vi "FTW-Test-SQLite-BasicQuery.vi"() -> (0 "Test Result":errorcluster)   [LabVIEW 2014]
uses:
  src/core/database/FTW-SQLite-DatabaseType.ctl
  src/core/time/FTW-Time-Uptime.vi
  src/core/error/FTW-ERR-Assert-DeveloperError.vi
  src/core/error/FTW-ERR-ThrowError.vi
  src/core/error/FTW-ERR-NoErrorConstant.vi
  src/core/database/FTW-SQLite-PrepareStatement.vi
  src/core/database/FTW-SQLite-LibraryReturnValue.vi
  src/core/error/FTW-ERR-CallChain.vi
  src/core/string/FTW-STR-ReplaceWhitespace.vi
  src/core/database/FTW-SQLite-Insert/FTW-SQLite-Insert.xnode
  src/core/database/FTW-SQLite-Connector.lvclass
  src/core/database/FTW-SQLite-Fetch/FTW-SQLite-Fetch.xnode
  src/core/database/FTW-SQLite-AccessMode.ctl
panel:
  out "Results from Database":T1(array[cluster])
  out "Data to put into Database":T2(array[cluster])
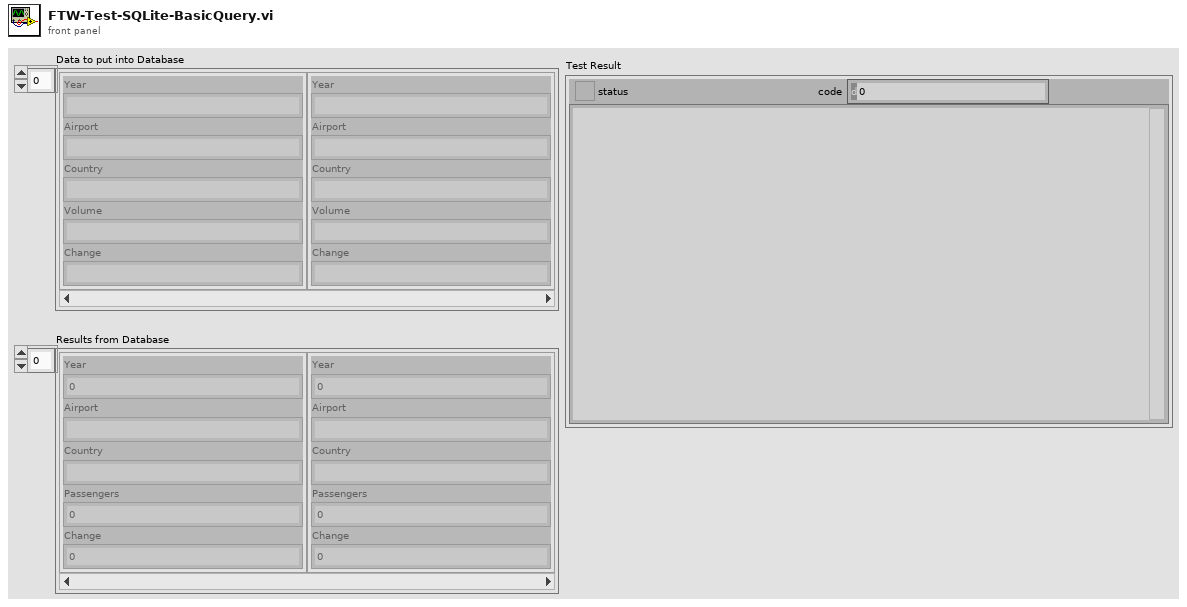
[diagram p1: front panel]
types:
  T1 = cluster{"Year":i32, "Airport":string, "Country":string, "Passengers":i32, "Change":dbl}[]
  T2 = cluster{"Year":string, "Airport":string, "Country":string, "Volume":string, "Change":string}[]
  T3 = cluster{"Year":string, "Airport":string, "Country":string, "Volume":string, "Change":string}
  T4 = cluster{"Year":i32, "Airport":string, "Country":string, "Passengers":i32, "Change":dbl}
  T5 = typedef "FTW-SQLite-Connector.lvclass/FTW-SQLite-DatabaseType.ctl" = enum16{"Disk", "Memory"}
  T6 = typedef "FTW-SQLite-Connector.lvclass/FTW-SQLite-AccessMode.ctl" = enum16{"Read", "Read/Write", "Read/Write/Create"}
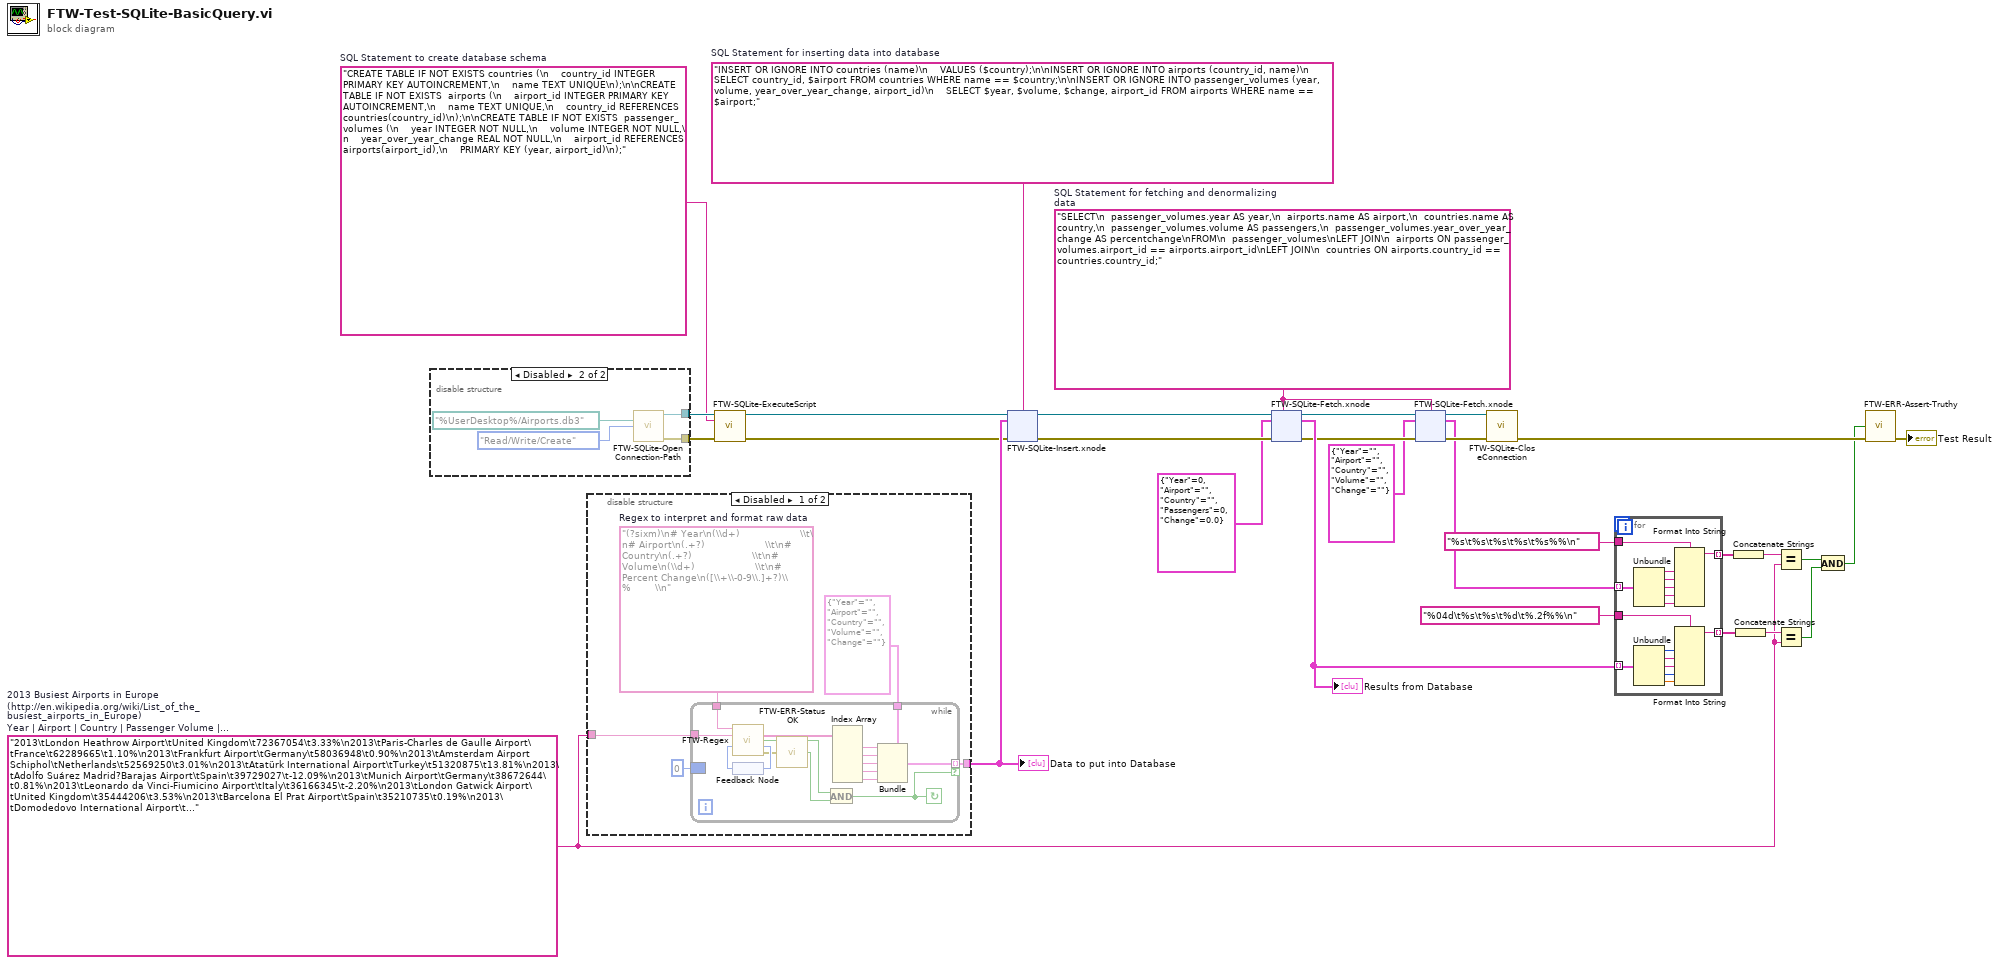
[diagram p0: block diagram]
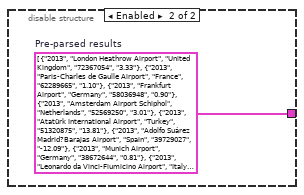
[diagram p2: hidden frame]
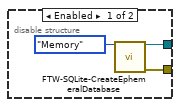
[diagram p3: hidden frame]
diagram:
  w23 = "INSERT OR IGNORE INTO countries (name)\n    VALUES ($country);\n\nINSERT OR IGNORE INTO airports (country_id, name)\n    SELECT country_id, $airport FROM countries WHERE name == $country;\n\nINSERT OR IGNORE INTO passenger_volumes (year, volume, year_over_year_change, airport_id)\n    SELECT $year, $volume, $change, airport_id FROM airports WHERE name == $airport;"  # SQL Statement for inserting data into database
  w10 = "SELECT\n  passenger_volumes.year AS year,\n  airports.name AS airport,\n  countries.name AS country,\n  passenger_volumes.volume AS passengers,\n  passenger_volumes.year_over_year_change AS percentchange\nFROM\n  passenger_volumes\nLEFT JOIN\n  airports ON passenger_volumes.airport_id == airports.airport_id\nLEFT JOIN\n  countries ON airports.country_id == countries.country_id;"  # SQL Statement for fetching and denormalizing data
  w2 = "2013\tLondon Heathrow Airport\tUnited Kingdom\t72367054\t3.33%\n2013\tParis-Charles de Gaulle Airport\tFrance\t62289665\t1.10%\n2013\tFrankfurt Airport\tGermany\t58036948\t0.90%\n2013\tAmsterdam Airport Schiphol\tNetherlands\t52569250\t3.01%\n2013\tAtatürk International Airport\tTurkey\t51320875\t13.81%\n2013\tAdolfo Suárez Madrid?Barajas Airport\tSpain\t39729027\t-12.09%\n2013\tMunich Airport\tGermany\t38672644\t0.81%\n2013\tLeonardo da Vinci-Fiumicino Airport\tItaly\t36166345\t-2.20%\n2013\tLondon Gatwick Airport\tUnited Kingdom\t35444206\t3.53%\n2013\tBarcelona El Prat Airport\tSpain\t35210735\t0.19%\n2013\tDomodedovo International Airport\tRussia\t30760000\t9.21%\n2013\tSheremetyevo International Airport\tRussia\t29256000\t12.38%\n2013\tParis-Orly Airport\tFrance\t28274154\t3.83%\n2013\tAntalya Airport\tTurkey\t27003712\t8.04%\n2013\tZürich Airport\tSwitzerland\t24865138\t0.25%\n2013\tCopenhagen Airport, Kastrup\tDenmark\t24067030\t3.13%\n2013\tOslo Gardermoen International Airport\tNorway\t22956540\t3.97%\n2013\tPalma de Mallorca Airport\tSpain\t22768082\t0.45%\n2013\tVienna International Airport\tAustria\t21999926\t-0.75%\n2013\tDüsseldorf International Airport\tGermany\t21228226\t1.90%\n2013\tManchester Airport\tUnited Kingdom\t20751581\t5.14%\n2013\tStockholm-Arlanda Airport\tSweden\t20681554\t5.29%\n2013\tDublin Airport\tIreland\t20200000\t5.76%\n2013\tBerlin Tegel Airport\tGermany\t19591838\t7.86%\n2013\tBrussels Airport\tBelgium\t19133222\t0.85%\n2013\tSabiha Gökçen Airport\tTurkey\t18641842\t28.68%\n2013\tMalpensa Airport\tItaly\t17955075\t-3.14%\n2013\tLondon Stansted Airport\tUnited Kingdom\t17852393\t2.17%\n2013\tLisbon Portela Airport\tPortugal\t16024955\t4.73%\n2013\tHelsinki-Vantaa Airport\tFinland\t15279043\t2.83%\n2013\tGeneva International Airport\tSwitzerland\t14436149\t3.86%\n2013\tHamburg Airport\tGermany\t13502553\t-1.42%\n2013\tMálaga Airport\tSpain\t12922403\t2.71%\n2013\tPulkovo Airport\tRussia\t12854366\t15.24%\n2013\tAthens International Airport\tGreece\t12460298\t-3.74%\n2013\tNice Côte d'Azur Airport\tFrance\t11554195\t3.26%\n2013\tVnukovo International Airport\tRussia\t11180000\t15.38%\n2013\tVáclav Havel Airport Prague\tCzech Republic\t10974196\t1.54%\n2013\tEsenbo?a International Airport\tTurkey\t10928403\t18.30%\n2013\tFrederic Chopin Airport\tPoland\t10683402\t11.43%\n2013\tAdnan Menderes Airport\tTurkey\t10208627\t9.11%\n2013\tEdinburgh Airport\tUnited Kingdom\t9775443\t6.31%\n2013\tGran Canaria Airport\tSpain\t9770253\t-1.23%\n2013\tLondon Luton Airport\tUnited Kingdom\t9697944\t0.83%\n2013\tAlicante Airport\tSpain\t9638860\t8.85%\n2013\tStuttgart Airport\tGermany\t9577551\t-1.47%\n2013\tBirmingham Airport\tUnited Kingdom\t9120201\t2.22%\n2013\tCologne Bonn Airport\tGermany\t9077346\t-2.18%\n2013\tLinate Airport\tItaly\t9034373\t-2.12%\n2013\tOrio al Serio Airport\tItaly\t8964376\t0.83%\n2013\tTenerife South Airport\tSpain\t8701983\t2.01%\n2013\tLyon-Saint Exupéry Airport\tFrance\t8562288\t1.32%\n2013\tBudapest Liszt Ferenc International Airport\tHungary\t8520880\t0.20%\n2013\tVenice Marco Polo Airport\tItaly\t8403790\t2.63%\n2013\tMarseille Provence Airport\tFrance\t8260619\t-0.42%\n2013\tBoryspil International Airport\tUkraine\t7930000\t-6.46%\n2013\tHenri Coand? International Airport\tRomania\t7649503\t7.44%\n2013\tBlagnac Airport\tFrance\t7567634\t0.11%\n2013\tGlasgow International Airport\tUnited Kingdom\t7363764\t2.88%\n2013\tBrussels South Charleroi Airport\tBelgium\t6786979\t4.15%\n2013\tBerlin Schönefeld Airport\tGermany\t6727306\t-5.21%\n2013\tCatania-Fontanarossa Airport\tItaly\t6400127\t2.45%\n2013\tFrancisco de Sá Carneiro Airport\tPortugal\t6370749\t5.30%\n2013\tBergen Flesland Airport\tNorway\t6213960\t6.87%\n2013\tBologna Airport\tItaly\t6193783\t3.95%\n2013\tBristol Airport\tUnited Kingdom\t6131896\t3.55%\n2013\tFaro Airport\tPortugal\t5978685\t5.40%\n2013\tEuroAirport Basel-Mulhouse-Freiburg\tSwitzerland-France-Germany\t5880771\t9.83%\n2013\tHeraklion International Airport\tGreece\t5792429\t15.52%\n2013\tIbiza Airport\tSpain\t5726581\t3.09%\n2013\tNaples Airport\tItaly\t5444422\t-6.16%\n2013\tLanzarote Airport\tSpain\t5334598\t3.21%\n2013\tLangenhagen Airport\tGermany\t5234909\t-1.00%\n2013\tGothenburg-Landvetter Airport\tSweden\t5004093\t3.07%\n2013\tLarnaca International Airport\tCyprus\t4863577\t-5.86%\n2013\tRiga International Airport\tLatvia\t4793213\t0.53%\n2013\tRome Ciampino Airport\tItaly\t4749251\t5.60%\n2013\tStavanger Sola Airport\tNorway\t4668403\t5.76%\n2013\tValencia Airport\tSpain\t4599990\t-3.20%\n2013\tBordeaux - Mérignac Airport\tFrance\t4574357\t4.43%\n2013\tGalileo Galilei Airport\tItaly\t4479690\t-0.34%\n2013\tNewcastle Airport\tUnited Kingdom\t4420839\t1.25%\n2013\tPalermo Airport\tItaly\t4349672\t-5.62%\n2013\tEast Midlands Airport\tUnited Kingdom\t4334117\t6.33%\n2013\tAdana ?akirpa?a Airport\tTurkey\t4316678\t14.28%\n2013\tTrondheim Værnes Airport\tNorway\t4311328\t3.63%\n2013\tKoltsovo Airport\tRussia\t4293002\t13.48%\n2013\tFuerteventura Airport\tSpain\t4259341\t-3.18%\n2013\tRhodes International Airport\tGreece\t4200068\t10.10%\n2013\tLiverpool John Lennon Airport\tUnited Kingdom\t4187493\t-6.18%\n2013\tThessaloniki International Airport, \"Macedonia\"\tGreece\t4085032\t1.05%\n2013\tDalaman Airport\tTurkey\t4057173\t6.49%\n2013\tMalta International Airport\tMalta\t4052000\t10.88%\n2013\tBelfast International Airport\tUnited Kingdom\t4023336\t-6.73%\n2013\tBeauvais-Tillé Airport\tFrance\t3952908\t2.34%\n2013\tNantes Atlantique Airport\tFrance\t3930849\t8.24%\n2013\tBilbao Airport\tSpain\t3800789\t-8.88%\n2013\tTolmachevo Airport\tRussia\t3748211\t14.74%\n2013\tSan Pablo Airport\tSpain\t3687727\t-14.08%\n2013\tKraków Airport\tPoland\t3647616\t6.07%\n2012\tLondon Heathrow Airport\tUnited Kingdom\t70037417\t0.87%\n2012\tParis-Charles de Gaulle Airport\tFrance\t61611934\t1.05%\n2012\tFrankfurt Airport\tGermany\t57520001\t1.92%\n2012\tAmsterdam Airport Schiphol\tNetherlands\t51035590\t2.57%\n2012\tMadrid?Barajas Airport\tSpain\t45190528\t-9.02%\n2012\tAtatürk International Airport\tTurkey\t45091962\t20.58%\n2012\tMunich Airport\tGermany\t38360604\t1.58%\n2012\tLeonardo da Vinci-Fiumicino Airport\tItaly\t36980911\t-1.78%\n2012\tBarcelona El Prat Airport\tSpain\t35144503\t2.17%\n2012\tLondon Gatwick Airport\tUnited Kingdom\t34235982\t1.67%\n2012\tDomodedovo International Airport\tRussia\t28165657\t9.59%\n2012\tParis-Orly Airport\tFrance\t27232263\t0.34%\n2012\tSheremetyevo International Airport\tRussia\t26032975\t16.47%\n2012\tAntalya Airport\tTurkey\t24993667\t-0.48%\n2012\tZürich Airport\tSwitzerland\t24802466\t1.91%\n2012\tCopenhagen Airport, Kastrup\tDenmark\t23336187\t2.69%\n2012\tPalma de Mallorca Airport\tSpain\t22666858\t-0.26%\n2012\tVienna International Airport\tAustria\t22165794\t5.02%\n2012\tOslo Gardermoen International Airport\tNorway\t22080433\t4.63%\n2012\tDüsseldorf International Airport\tGermany\t20833246\t2.43%\n2012\tManchester Airport\tUnited Kingdom\t19736502\t4.47%\n2012\tStockholm-Arlanda Airport\tSweden\t19642029\t3.00%\n2012\tDublin Airport\tIreland\t19099649\t1.91%\n2012\tBrussels Airport\tBelgium\t18971332\t0.99%\n2012\tMalpensa Airport\tItaly\t18537301\t-3.97%\n2012\tBerlin Tegel Airport\tGermany\t18164203\t7.35%\n2012\tLondon Stansted Airport\tUnited Kingdom\t17472699\t-3.21%\n2012\tLisbon Portela Airport\tPortugal\t15301176\t3.35%\n2012\tHelsinki Airport\tFinland\t14858215\t-0.05%\n2012\tSabiha Gökçen Airport\tTurkey\t14487242\t13.63%\n2012\tGeneva International Airport\tSwitzerland\t13899422\t6.01%\n2012\tHamburg Airport\tGermany\t13697402\t1.03%\n2012\tAthens International Airport\tGreece\t12944041\t-10.40%\n2012\tMálaga Airport\tSpain\t12581944\t-1.88%\n2012\tNice Côte d'Azur Airport\tFrance\t11189896\t7.37%\n2012\tPulkovo Airport\tRussia\t11154560\t16.06%\n2012\tVáclav Havel Airport Prague\tCzech Republic\t10807890\t-8.32%\n2012\tGran Canaria Airport\tSpain\t9892067\t-6.14%\n2012\tStuttgart Airport\tGermany\t9720877\t1.45%\n2012\tVnukovo International Airport\tRussia\t9690000\t18.21%\n2012\tLondon Luton Airport\tUnited Kingdom\t9617697\t1.09%\n2012\tFrederic Chopin Airport\tPoland\t9587842\t2.68%\n2012\tAdnan Menderes Airport\tTurkey\t9356284\t9.77%\n2012\tCologne Bonn Airport\tGermany\t9280070\t-3.57%\n2012\tEsenbo?a Airport\tTurkey\t9237886\t8.87%\n2012\tLinate Airport\tItaly\t9229890\t1.11%\n2012\tEdinburgh Airport\tUnited Kingdom\t9195061\t-2.03%\n2012\tBirmingham Airport\tUnited Kingdom\t8922539\t3.55%\n2012\tOrio al Serio Airport\tItaly\t8890720\t5.59%\n2012\tAlicante Airport\tSpain\t8855444\t-10.67%\n2012\tTenerife South Airport\tSpain\t8530729\t-1.45%\n2012\tBudapest Liszt Ferenc International Airport\tHungary\t8504020\t-4.67%\n2012\tBoryspil International Airport\tUkraine\t8478091\t5.36%\n2012\tLyon-Saint Exupéry Airport\tFrance\t8451039\t0.16%\n2012\tMarseille Provence Airport\tFrance\t8295479\t12.61%\n2012\tVenice Marco Polo Airport\tItaly\t8188455\t-4.62%\n2012\tBlagnac Airport\tFrance\t7559350\t8.17%\n2012\tGlasgow International Airport\tUnited Kingdom\t7157859\t4.04%\n2012\tHenri Coand? International Airport\tRomania\t7120067\t41.01%\n2012\tBerlin Schönefeld Airport\tGermany\t7097274\t-0.23%\n2012\tBrussels South Charleroi Airport\tBelgium\t6516427\t10.43%\n2012\tCatania-Fontanarossa Airport\tItaly\t6246888\t-8.05%\n2012\tFrancisco de Sá Carneiro Airport\tPortugal\t6050094\t0.76%\n2012\tBologna Airport\tItaly\t5958648\t1.24%\n2012\tBristol Airport\tUnited Kingdom\t5921530\t2.44%\n2012\tBergen Flesland Airport\tNorway\t5814413\t3.80%\n2012\tNaples Airport\tItaly\t5801836\t0.57%\n2012\tFaro Airport\tPortugal\t5672377\t1.01%\n2012\tIbiza Airport\tSpain\t5555048\t-1.56%\n2012\tEuroAirport Basel-Mulhouse-Freiburg\tSwitzerland-France-Germany\t5354674\t5.96%\n2012\tLangenhagen Airport\tGermany\t5287831\t-0.98%\n2012\tLanzarote Airport\tSpain\t5168775\t-6.76%\n2012\tLarnaca International Airport\tCyprus\t5166224\t-6.20%\n2012\tHeraklion International Airport\tGreece\t5014312\t-5.26%\n2012\tGothenburg-Landvetter Airport\tSweden\t4854888\t-1.05%\n2012\tRiga International Airport\tLatvia\t4767878\t-6.64%\n2012\tValencia Airport\tSpain\t4752020\t-4.57%\n2012\tPalermo Airport\tItaly\t4608533\t-7.70%\n2012\tRome Ciampino Airport\tItaly\t4497376\t-5.95%\n2012\tGalileo Galilei Airport\tItaly\t4494915\t-0.70%\n2012\tLiverpool John Lennon Airport\tUnited Kingdom\t4463257\t-15.00%\n2012\tStavanger Sola Airport\tNorway\t4413987\t6.83%\n2012\tFuerteventura Airport\tSpain\t4399023\t-11.10%\n2012\tBordeaux - Mérignac Airport\tFrance\t4380145\t6.38%\n2012\tNewcastle Airport\tUnited Kingdom\t4366196\t0.46%\n2012\tBelfast International Airport\tUnited Kingdom\t4313685\t5.12%\n2012\tSan Pablo Airport\tSpain\t4292020\t-13.46%\n2012\tBilbao Airport\tSpain\t4171065\t3.09%\n2012\tTrondheim Værnes Airport\tNorway\t4160162\t5.95%\n2012\tEast Midlands Airport\tUnited Kingdom\t4076178\t-3.30%\n2012\tThessaloniki International Airport, \"Macedonia\"\tGreece\t4042539\t-0.47%\n2012\tBeauvais-Tillé Airport\tFrance\t3862431\t5.02%\n2012\tRhodes International Airport\tGreece\t3814706\t-8.06%\n2012\tDalaman Airport\tTurkey\t3810015\t2.06%\n2012\tKoltsovo Airport\tRussia\t3783069\t12.73%\n2012\tBari Airport\tItaly\t3780112\t1.46%\n2012\tAdana ?akirpa?a Airport\tTurkey\t3777348\t16.55%\n2012\tLos Rodeos Airport\tSpain\t3717944\t-9.21%\n2012\tMalta International Airport\tMalta\t3654283\t4.10%\n2012\tNantes Atlantique Airport\tFrance\t3631693\t11.88%\n2011\tLondon Heathrow Airport\tUnited Kingdom\t69433230\t5.39%\n2011\tParis-Charles de Gaulle Airport\tFrance\t60970551\t4.82%\n2011\tFrankfurt Airport\tGermany\t56436255\t6.46%\n2011\tAmsterdam Airport Schiphol\tNetherlands\t49755252\t10.05%\n2011\tMadrid Barajas Airport\tSpain\t49671270\t-0.39%\n2011\tMunich Airport\tGermany\t37763701\t8.76%\n2011\tRome-Fiumicino Airport\tItaly\t37651700\t3.62%\n2011\tAtatürk International Airport\tTurkey\t37394694\t16.34%\n2011\tBarcelona El Prat Airport\tSpain\t34398226\t17.76%\n2011\tLondon Gatwick Airport\tUnited Kingdom\t33674264\t7.33%\n2011\tParis-Orly Airport\tFrance\t27139076\t7.68%\n2011\tDomodedovo International Airport\tRussia\t25701610\t15.49%\n2011\tAntalya Airport\tTurkey\t25113635\t14.09%\n2011\tZurich Airport\tSwitzerland\t24337954\t6.38%\n2011\tPalma de Mallorca Airport\tSpain\t22726707\t7.62%\n2011\tCopenhagen Airport\tDenmark\t22725517\t5.69%\n2011\tSheremetyevo International Airport\tRussia\t22351317\t16.88%\n2011\tVienna International Airport\tAustria\t21106292\t7.19%\n2011\tOslo-Gardermoen Airport\tNorway\t21103623\t10.54%\n2011\tDüsseldorf International Airport\tGermany\t20339466\t7.12%\n2011\tMilan Malpensa Airport\tItaly\t19303131\t1.88%\n2011\tStockholm-Arlanda Airport\tSweden\t19069065\t12.42%\n2011\tManchester Airport\tUnited Kingdom\t18892756\t6.38%\n2011\tBrussels Airport\tBelgium\t18786034\t9.34%\n2011\tDublin Airport\tIreland\t18740593\t1.68%\n2011\tLondon Stansted Airport\tUnited Kingdom\t18052843\t-2.80%\n2011\tBerlin Tegel Airport\tGermany\t16919820\t12.61%\n2011\tHelsinki Airport\tFinland\t14865871\t15.39%\n2011\tLisbon Portela Airport\tPortugal\t14805624\t5.49%\n2011\tAthens International Airport\tGreece\t14446963\t-5.59%\n2011\tHamburg Airport\tGermany\t13558261\t4.60%\n2011\tGeneva Cointrin International Airport\tSwitzerland\t13111741\t11.25%\n2011\tMálaga Airport\tSpain\t12823117\t6.29%\n2011\tSabiha Gökçen Airport\tTurkey\t12749230\t13.94%\n2011\tVáclav Havel Airport Prague\tCzech Republic\t11788629\t2.01%\n2011\tGran Canaria Airport\tSpain\t10538829\t11.10%\n2011\tNice Côte d'Azur Airport\tFrance\t10422073\t8.53%\n2011\tAlicante Airport\tSpain\t9913731\t5.66%\n2011\tCologne Bonn Airport\tGermany\t9623398\t-2.30%\n2011\tPulkovo Airport\tRussia\t9610767\t14.53%\n2011\tStuttgart Airport\tGermany\t9582265\t3.95%\n2011\tLondon Luton Airport\tUnited Kingdom\t9513704\t8.87%\n2011\tEdinburgh Airport\tUnited Kingdom\t9385245\t9.17%\n2011\tFrederic Chopin Airport\tPoland\t9337734\t7.18%\n2011\tMilan Linate Airport\tItaly\t9128522\t10.03%\n2011\tBudapest Liszt Ferenc International Airport\tHungary\t8920653\t8.92%\n2011\tTenerife South Airport\tSpain\t8656487\t17.63%\n2011\tBirmingham Airport\tUnited Kingdom\t8616296\t0.51%\n2011\tVenice Marco Polo Airport\tItaly\t8584651\t25.24%\n2011\tAdnan Menderes Airport\tTurkey\t8523533\t13.87%\n2011\tEsenbo?a Airport\tTurkey\t8485467\t9.29%\n2011\tLyon-Saint Exupéry Airport\tFrance\t8437141\t5.74%\n2011\tBergamo Orio al Serio airport\tItaly\t8419948\t9.67%\n2011\tVnukovo International Airport\tRussia\t8197162\t-13.35%\n2011\tBoryspil International Airport\tUkraine\t8047115\t20.24%\n2011\tMarseille Provence Airport\tFrance\t7366873\t-2.10%\n2011\tBerlin Schönefeld Airport\tGermany\t7113989\t-2.52%\n2011\tBlagnac Airport\tFrance\t6988140\t9.09%\n2011\tGlasgow International Airport\tUnited Kingdom\t6880217\t5.06%\n2011\tCatania-Fontanarossa Airport\tItaly\t6794063\t7.53%\n2011\tFrancisco de Sá Carneiro Airport\tPortugal\t6004589\t13.74%\n2011\tBrussels South Charleroi Airport\tBelgium\t5901007\t13.58%\n2011\tBologna Airport\tItaly\t5885884\t6.96%\n2011\tBristol Airport\tUnited Kingdom\t5780746\t0.58%\n2011\tNaples Airport\tItaly\t5768873\t3.54%\n2011\tIbiza Airport\tSpain\t5643180\t11.95%\n2011\tFaro Airport\tPortugal\t5615580\t5.24%\n2011\tBergen Airport\tNorway\t5814413\t14.50%\n2011\tLanzarote Airport\tSpain\t5543744\t12.26%\n2011\tLarnaca International Airport\tCyprus\t5507762\t2.61%\n2011\tLangenhagen Airport\tGermany\t5340264\t5.54%\n2011\tHeraklion International Airport\tGreece\t5292687\t7.85%\n2011\tLiverpool John Lennon Airport\tUnited Kingdom\t5251161\t4.73%\n2011\tRiga International Airport\tLatvia\t5106926\t9.50%\n2011\tEuroAirport Basel-Mulhouse-Freiburg\tSwitzerland-France-Germany\t5053664\t22.39%\n2011\tHenri Coand? International Airport\tRomania\t5049443\t2.67%\n2011\tPalermo Airport\tItaly\t4992798\t14.96%\n2011\tValencia Airport\tSpain\t4979511\t0.92%\n2011\tSan Pablo Airport\tSpain\t4959359\t17.39%\n2011\tFuerteventura Airport\tSpain\t4948018\t18.56%\n2011\tGothenburg-Landvetter Airport\tSweden\t4906639\t18.71%\n2011\tRome Ciampino Airport\tItaly\t4781731\t5.51%\n2011\tPisa Airport\tItaly\t4526723\t11.52%\n2011\tNewcastle Airport\tUnited Kingdom\t4346270\t-0.23%\n2011\tEast Midlands Airport\tUnited Kingdom\t4215192\t2.47%\n2011\tRhodes International Airport\tGreece\t4149274\t15.69%\n2011\tStavanger Airport\tNorway\t4131974\t12.44%\n2011\tBordeaux - Mérignac Airport\tFrance\t4117303\t12.38%\n2011\tBelfast International Airport\tUnited Kingdom\t4103620\t2.18%\n2011\tLos Rodeos Airport\tSpain\t4095103\t1.08%\n2011\tThessaloniki International Airport, \"Macedonia\"\tGreece\t4061697\t3.86%\n2011\tBilbao Airport\tSpain\t4046172\t4.04%\n2011\tNuremberg Airport\tGermany\t3962617\t-2.61%\n2011\tTrondheim Airport\tNorway\t3926461\t11.49%\n2011\tDalaman Airport\tTurkey\t3732941\t-1.40%\n2011\tBari Airport\tItaly\t3725629\t9.64%\n2011\tTurin Airport\tItaly\t3710485\t4.45%\n2011\tCagliari-Elmas Airport\tItaly\t3698982\t7.43%\n2011\tBeauvais-Tillé Airport\tFrance\t3677825\t25.45%\n2011\tMalta International Airport\tMalta\t3510213\t6.36%\n2010\tLondon Heathrow Airport\tUnited Kingdom\t65881660\t-0.24%\n2010\tParis-Charles de Gaulle Airport\tFrance\t58164612\t0.45%\n2010\tFrankfurt Airport\tGermany\t53009221\t4.08%\n2010\tBarajas Airport\tSpain\t49866113\t2.95%\n2010\tAmsterdam Airport Schiphol\tNetherlands\t45211749\t3.77%\n2010\tLeonardo da Vinci-Fiumicino Airport\tItaly\t36337050\t7.48%\n2010\tMunich Airport\tGermany\t34721605\t6.24%\n2010\tAtatürk International Airport\tTurkey\t32143819\t7.82%\n2010\tGatwick Airport\tUnited Kingdom\t31375290\t-3.14%\n2010\tBarcelona El Prat Airport\tSpain\t29209536\t6.52%\n2010\tParis-Orly Airport\tFrance\t25203969\t0.38%\n2010\tZurich Airport\tSwitzerland\t22878251\t4.34%\n2010\tDomodedovo International Airport\tRussia\t22253529\t19.16%\n2010\tAntalya Airport\tTurkey\t22013027\t19.99%\n2010\tCopenhagen Airport\tDenmark\t21501750\t9.06%\n2010\tPalma de Mallorca Airport\tSpain\t21117417\t-0.40%\n2010\tVienna International Airport\tAustria\t19691206\t8.71%\n2010\tSheremetyevo International Airport\tRussia\t19123007\t29.52%\n2010\tOslo-Gardermoen Airport\tNorway\t19091036\t5.55%\n2010\tDüsseldorf International Airport\tGermany\t18988149\t6.71%\n2010\tMalpensa Airport\tItaly\t18947808\t7.95%\n2010\tLondon Stansted Airport\tUnited Kingdom\t18573592\t-6.93%\n2010\tDublin Airport\tIreland\t18431064\t-10.11%\n2010\tManchester Airport\tUnited Kingdom\t17759173\t-5.16%\n2010\tBrussels Airport\tBelgium\t17180606\t1.07%\n2010\tStockholm-Arlanda Airport\tSweden\t16962416\t5.59%\n2010\tAthens International Airport\tGreece\t15303127\t-5.69%\n2010\tBerlin Tegel Airport\tGermany\t15025600\t5.96%\n2010\tLisbon Portela Airport\tPortugal\t14035273\t5.70%\n2010\tHamburg Airport\tGermany\t12962429\t5.99%\n2010\tHelsinki Airport\tFinland\t12883399\t2.32%\n2010\tMálaga Airport\tSpain\t12064521\t3.80%\n2010\tGeneva Cointrin International Airport\tSwitzerland\t11785522\t4.07%\n2010\tRuzyn? Airport\tCzech Republic\t11556858\t-0.74%\n2010\tSabiha Gökçen Airport\tTurkey\t11189678\t68.51%\n2010\tCologne Bonn Airport\tGermany\t9849779\t1.13%\n2010\tNice Côte d'Azur Airport\tFrance\t9603014\t-2.32%\n2010\tGran Canaria Airport\tSpain\t9486035\t3.61%\n2010\tVnukovo International Airport\tRussia\t9460292\t22.37%\n2010\tAlicante Airport\tSpain\t9382931\t2.66%\n2010\tStuttgart Airport\tGermany\t9218095\t3.17%\n2010\tLondon Luton Airport\tUnited Kingdom\t8738712\t-4.19%\n2010\tFrederic Chopin Airport\tPoland\t8712384\t4.70%\n2010\tEdinburgh Airport\tUnited Kingdom\t8596715\t-5.00%\n2010\tBirmingham Airport\tUnited Kingdom\t8572398\t-5.83%\n2010\tPulkovo Airport\tRussia\t8391281\t24.17%\n2010\tLinate Airport\tItaly\t8296450\t0.02%\n2010\tBudapest Liszt Ferenc International Airport\tHungary\t8190089\t1.17%\n2010\tLyon-Saint Exupéry Airport\tFrance\t7979228\t3.39%\n2010\tEsenbo?a Airport\tTurkey\t7763914\t27.60%\n2010\tOrio al Serio Airport\tItaly\t7677224\t7.26%\n2010\tMarseille Provence Airport\tFrance\t7524886\t3.22%\n2010\tAdnan Menderes Airport\tTurkey\t7485098\t20.69%\n2010\tTenerife South Airport\tSpain\t7358986\t3.53%\n2010\tBerlin Schönefeld Airport\tGermany\t7297911\t7.37%\n2010\tVenice Marco Polo Airport\tItaly\t6854595\t2.28%\n2010\tBoryspil International Airport\tUkraine\t6692382\t15.49%\n2010\tGlasgow International Airport\tUnited Kingdom\t6548865\t-9.36%\n2010\tBlagnac Airport\tFrance\t6405906\t2.04%\n2010\tCatania-Fontanarossa Airport\tItaly\t6318177\t6.52%\n2010\tBristol Airport\tUnited Kingdom\t5747604\t1.86%\n2010\tNaples Airport\tItaly\t5571738\t4.91%\n2010\tBologna Airport\tItaly\t5503106\t15.26%\n2010\tLarnaca International Airport\tCyprus\t5367724\t3.85%\n2010\tFaro Airport\tPortugal\t5336173\t5.31%\n2010\tFrancisco de Sá Carneiro Airport\tPortugal\t5279362\t17.08%\n2010\tBrussels South Charleroi Airport\tBelgium\t5195372\t31.96%\n2010\tBergen Airport\tNorway\t5078267\t4.43%\n2010\tLangenhagen Airport\tGermany\t5059800\t1.81%\n2010\tIbiza Airport\tSpain\t5040800\t10.23%\n2010\tLiverpool John Lennon Airport\tUnited Kingdom\t5013940\t2.65%\n2010\tLanzarote Airport\tSpain\t4938343\t5.03%\n2010\tValencia Airport\tSpain\t4934268\t3.90%\n2010\tHenri Coand? International Airport\tRomania\t4917952\t9.69%\n2010\tHeraklion International Airport\tGreece\t4907337\t-2.88%\n2010\tGirona-Costa Brava Airport\tSpain\t4863954\t-8.00%\n2010\tRiga International Airport\tLatvia\t4663647\t14.67%\n2010\tRome Ciampino Airport\tItaly\t4531834\t-4.75%\n2010\tNewcastle Airport\tUnited Kingdom\t4356130\t-5.05%\n2010\tPalermo Airport\tItaly\t4343227\t-0.17%\n2010\tSan Pablo Airport\tSpain\t4224718\t4.28%\n2010\tFuerteventura Airport\tSpain\t4173590\t11.64%\n2010\tGothenburg-Landvetter Airport\tSweden\t4133299\t12.04%\n2010\tEuroAirport Basel-Mulhouse-Freiburg\tSwitzerland-France-Germany\t4129186\t7.24%\n2010\tEast Midlands Airport\tUnited Kingdom\t4113501\t-11.69%\n2010\tNuremberg Airport\tGermany\t4068799\t2.60%\n2010\tGalileo Galilei Airport\tItaly\t4058957\t1.18%\n2010\tLos Rodeos Airport\tSpain\t4051356\t-0.07%\n2010\tBelfast International Airport\tUnited Kingdom\t4016170\t-11.66%\n2010\tThessaloniki International Airport, \"Macedonia\"\tGreece\t3910751\t-4.71%\n2010\tBilbao Airport\tSpain\t3888955\t6.40%\n2010\tDalaman Airport\tTurkey\t3785779\t5.22%\n2010\tStavanger Airport\tNorway\t3674816\t1.57%\n2010\tBordeaux - Mérignac Airport\tFrance\t3663702\t10.42%\n2010\tRhodes International Airport\tGreece\t3586572\t3.36%\n2010\tTurin Airport\tItaly\t3552519\t10.31%\n2010\tTrondheim Airport\tNorway\t3521734\t2.83%\n2010\tFrankfurt-Hahn Airport\tGermany\t3493451\t-7.91%\n2010\tCagliari-Elmas Airport\tItaly\t3438298\t3.28%\n2010\tBari Airport\tItaly\t3398110\t20.27%\n"  # 2013 Busiest Airports in Europe (http://en.wikipedia.org/wiki/List_of_the_busiest_airports_in_Europe) Year | Airport | Country | Passenger Volume | Percent Change over Previous Year
  w28 = "CREATE TABLE IF NOT EXISTS countries (\n    country_id INTEGER PRIMARY KEY AUTOINCREMENT,\n    name TEXT UNIQUE\n);\n\nCREATE TABLE IF NOT EXISTS  airports (\n    airport_id INTEGER PRIMARY KEY AUTOINCREMENT,\n    name TEXT UNIQUE,\n    country_id REFERENCES countries(country_id)\n);\n\nCREATE TABLE IF NOT EXISTS  passenger_volumes (\n    year INTEGER NOT NULL,\n    volume INTEGER NOT NULL,\n    year_over_year_change REAL NOT NULL,\n    airport_id REFERENCES airports(airport_id),\n    PRIMARY KEY (year, airport_id)\n);"  # SQL Statement to create database schema
  n1 = disable-structure shown="Disabled" {
    disable-tunnel: [w32 w36] -> w30
    disable-tunnel: [w31 w37] -> w29
    frame Enabled {
      n2 = call "FTW-SQLite-CreateEphemeralDatabase.vi"("Database Type"=FTW-SQLite-DatabaseType."Memory") -> ("SQLite Connector"=w31:refnum<class "FTW-SQLite-Connector.lvclass">, "error out"=w32:errorcluster)  [unwired: 13 in]
    }
    frame Disabled {
      n3 = call "FTW-SQLite-OpenConnection-Path.vi"("Database Filepath"=path "%UserDesktop%/Airports.db3", "Access Mode"=FTW-SQLite-AccessMode."Read/Write/Create") -> ("SQLite Connector"=w37:refnum<class "FTW-SQLite-Connector.lvclass">, "error out"=w36:errorcluster)  [unwired: 12 in]
    }
  }
  n4 = disable-structure shown="Disabled" {
    disable-tunnel: w2 -> [w39 _]
    disable-tunnel: [w38 w59] -> w22
    frame Disabled {
      w42 = "(?sixm)\n# Year\n(\\d+)                    \\t\n# Airport\n(.+?)                    \\t\n# Country\n(.+?)                    \\t\n# Volume\n(\\d+)                    \\t\n# Percent Change\n([\\+\\-0-9\\.]+?)\\%        \\n"  # Regex to interpret and format raw data
      n5 = while {
        tunnel: w39 -> [w58]
        tunnel: T3 {"Year"="", "Airport"="", "Country"="", "Volume"="", "Change"=""} -> [w54]
        tunnel: w42 -> [w48]
        border: 0 ("Offset after Match") -> [_]
        tunnel: [w46] -> w38 mode=indexing if=w43
        stop <- w43 continue-if-true
        n6 = feedback #1() -> (w57:i32)
        n7 = call "FTW-Regex.vi"("Regular Expression"=w48, "Input String"=w58, "Starting Offset"=w57) -> ("Submatches"=w55:string[], "Match Found?"=w45:bool, "Offset after Match"=w56:i32, "error out"=w44:errorcluster)  [unwired: 8 in, 1 out]
        n8 = feedback-in #1(w56) -> ()
        n9 = call "FTW-ERR-StatusOK.vi"("error to check"=w44) -> ("Status OK?"=w47:bool)
        n10 = And(x=w45, y=w47) -> (x .and. y?=w43:bool)
        n11 = Index Array(array=w55) -> (element #1=w53:string, element #2=w52:string, element #3=w51:string, element #4=w50:string, element #5=w49:string)  [unwired: 5 in]
        n12 = Bundle(cluster=w54, "Year"=w53, "Airport"=w52, "Country"=w51, "Volume"=w50, "Change"=w49) -> (w46:T3)
      }
    }
    frame Enabled {
      w59 = T2 [{"Year"="2013", "Airport"="London Heathrow Airport", "Country"="United Kingdom", "Volume"="72367054", "Change"="3.33"}, {"Year"="2013", "Airport"="Paris-Charles de Gaulle Airport", "Country"="France", "Volume"="62289665", "Change"="1.10"}, {"Year"="2013", "Airport"="Frankfurt Airport", "Country"="Germany", "Volume"="58036948", "Change"="0.90"}, {"Year"="2013", "Airport"="Amsterdam Airport Schiphol", "Country"="Netherlands", "Volume"="52569250", "Change"="3.01"}, {"Year"="2013", "Airport"="Atatürk International Airport", "Country"="Turkey", "Volume"="51320875", "Change"="13.81"}, {"Year"="2013", "Airport"="Adolfo Suárez Madrid?Barajas Airport", "Country"="Spain", "Volume"="39729027", "Change"="-12.09"}, {"Year"="2013", "Airport"="Munich Airport", "Country"="Germany", "Volume"="38672644", "Change"="0.81"}, {"Year"="2013", "Airport"="Leonardo da Vinci-Fiumicino Airport", "Country"="Italy", "Volume"="36166345", "Change"="-2.20"}, {"Year"="2013", "Airport"="London Gatwick Airport", "Country"="United Kingdom", "Volume"="35444206", "Change"="3.53"}, {"Year"="2013", "Airport"="Barcelona El Prat Airport", "Country"="Spain", "Volume"="35210735", "Change"="0.19"}, {"Year"="2013", "Airport"="Domodedovo International Airport", "Country"="Russia", "Volume"="30760000", "Change"="9.21"}, {"Year"="2013", "Airport"="Sheremetyevo International Airport", "Country"="Russia", "Volume"="29256000", "Change"="12.38"}, {"Year"="2013", "Airport"="Paris-Orly Airport", "Country"="France", "Volume"="28274154", "Change"="3.83"}, {"Year"="2013", "Airport"="Antalya Airport", "Country"="Turkey", "Volume"="27003712", "Change"="8.04"}, {"Year"="2013", "Airport"="Zürich Airport", "Country"="Switzerland", "Volume"="24865138", "Change"="0.25"}, {"Year"="2013", "Airport"="Copenhagen Airport, Kastrup", "Country"="Denmark", "Volume"="24067030", "Change"="3.13"}, {"Year"="2013", "Airport"="Oslo Gardermoen International Airport", "Country"="Norway", "Volume"="22956540", "Change"="3.97"}, {"Year"="2013", "Airport"="Palma de Mallorca Airport", "Country"="Spain", "Volume"="22768082", "Change"="0.45"}, {"Year"="2013", "Airport"="Vienna International Airport", "Country"="Austria", "Volume"="21999926", "Change"="-0.75"}, {"Year"="2013", "Airport"="Düsseldorf International Airport", "Country"="Germany", "Volume"="21228226", "Change"="1.90"}, {"Year"="2013", "Airport"="Manchester Airport", "Country"="United Kingdom", "Volume"="20751581", "Change"="5.14"}, {"Year"="2013", "Airport"="Stockholm-Arlanda Airport", "Country"="Sweden", "Volume"="20681554", "Change"="5.29"}, {"Year"="2013", "Airport"="Dublin Airport", "Country"="Ireland", "Volume"="20200000", "Change"="5.76"}, {"Year"="2013", "Airport"="Berlin Tegel Airport", "Country"="Germany", "Volume"="19591838", "Change"="7.86"}, {"Year"="2013", "Airport"="Brussels Airport", "Country"="Belgium", "Volume"="19133222", "Change"="0.85"}, {"Year"="2013", "Airport"="Sabiha Gökçen Airport", "Country"="Turkey", "Volume"="18641842", "Change"="28.68"}, {"Year"="2013", "Airport"="Malpensa Airport", "Country"="Italy", "Volume"="17955075", "Change"="-3.14"}, {"Year"="2013", "Airport"="London Stansted Airport", "Country"="United Kingdom", "Volume"="17852393", "Change"="2.17"}, {"Year"="2013", "Airport"="Lisbon Portela Airport", "Country"="Portugal", "Volume"="16024955", "Change"="4.73"}, {"Year"="2013", "Airport"="Helsinki-Vantaa Airport", "Country"="Finland", "Volume"="15279043", "Change"="2.83"}, {"Year"="2013", "Airport"="Geneva International Airport", "Country"="Switzerland", "Volume"="14436149", "Change"="3.86"}, {"Year"="2013", "Airport"="Hamburg Airport", "Country"="Germany", "Volume"="13502553", "Change"="-1.42"}, {"Year"="2013", "Airport"="Málaga Airport", "Country"="Spain", "Volume"="12922403", "Change"="2.71"}, {"Year"="2013", "Airport"="Pulkovo Airport", "Country"="Russia", "Volume"="12854366", "Change"="15.24"}, {"Year"="2013", "Airport"="Athens International Airport", "Country"="Greece", "Volume"="12460298", "Change"="-3.74"}, {"Year"="2013", "Airport"="Nice Côte d'Azur Airport", "Country"="France", "Volume"="11554195", "Change"="3.26"}, {"Year"="2013", "Airport"="Vnukovo International Airport", "Country"="Russia", "Volume"="11180000", "Change"="15.38"}, {"Year"="2013", "Airport"="Václav Havel Airport Prague", "Country"="Czech Republic", "Volume"="10974196", "Change"="1.54"}, {"Year"="2013", "Airport"="Esenbo?a International Airport", "Country"="Turkey", "Volume"="10928403", "Change"="18.30"}, {"Year"="2013", "Airport"="Frederic Chopin Airport", "Country"="Poland", "Volume"="10683402", "Change"="11.43"}, {"Year"="2013", "Airport"="Adnan Menderes Airport", "Country"="Turkey", "Volume"="10208627", "Change"="9.11"}, {"Year"="2013", "Airport"="Edinburgh Airport", "Country"="United Kingdom", "Volume"="9775443", "Change"="6.31"}, {"Year"="2013", "Airport"="Gran Canaria Airport", "Country"="Spain", "Volume"="9770253", "Change"="-1.23"}, {"Year"="2013", "Airport"="London Luton Airport", "Country"="United Kingdom", "Volume"="9697944", "Change"="0.83"}, {"Year"="2013", "Airport"="Alicante Airport", "Country"="Spain", "Volume"="9638860", "Change"="8.85"}, {"Year"="2013", "Airport"="Stuttgart Airport", "Country"="Germany", "Volume"="9577551", "Change"="-1.47"}, {"Year"="2013", "Airport"="Birmingham Airport", "Country"="United Kingdom", "Volume"="9120201", "Change"="2.22"}, {"Year"="2013", "Airport"="Cologne Bonn Airport", "Country"="Germany", "Volume"="9077346", "Change"="-2.18"}, {"Year"="2013", "Airport"="Linate Airport", "Country"="Italy", "Volume"="9034373", "Change"="-2.12"}, {"Year"="2013", "Airport"="Orio al Serio Airport", "Country"="Italy", "Volume"="8964376", "Change"="0.83"}, {"Year"="2013", "Airport"="Tenerife South Airport", "Country"="Spain", "Volume"="8701983", "Change"="2.01"}, {"Year"="2013", "Airport"="Lyon-Saint Exupéry Airport", "Country"="France", "Volume"="8562288", "Change"="1.32"}, {"Year"="2013", "Airport"="Budapest Liszt Ferenc International Airport", "Country"="Hungary", "Volume"="8520880", "Change"="0.20"}, {"Year"="2013", "Airport"="Venice Marco Polo Airport", "Country"="Italy", "Volume"="8403790", "Change"="2.63"}, {"Year"="2013", "Airport"="Marseille Provence Airport", "Country"="France", "Volume"="8260619", "Change"="-0.42"}, {"Year"="2013", "Airport"="Boryspil International Airport", "Country"="Ukraine", "Volume"="7930000", "Change"="-6.46"}, {"Year"="2013", "Airport"="Henri Coand? International Airport", "Country"="Romania", "Volume"="7649503", "Change"="7.44"}, {"Year"="2013", "Airport"="Blagnac Airport", "Country"="France", "Volume"="7567634", "Change"="0.11"}, {"Year"="2013", "Airport"="Glasgow International Airport", "Country"="United Kingdom", "Volume"="7363764", "Change"="2.88"}, {"Year"="2013", "Airport"="Brussels South Charleroi Airport", "Country"="Belgium", "Volume"="6786979", "Change"="4.15"}, {"Year"="2013", "Airport"="Berlin Schönefeld Airport", "Country"="Germany", "Volume"="6727306", "Change"="-5.21"}, {"Year"="2013", "Airport"="Catania-Fontanarossa Airport", "Country"="Italy", "Volume"="6400127", "Change"="2.45"}, {"Year"="2013", "Airport"="Francisco de Sá Carneiro Airport", "Country"="Portugal", "Volume"="6370749", "Change"="5.30"}, {"Year"="2013", "Airport"="Bergen Flesland Airport", "Country"="Norway", "Volume"="6213960", "Change"="6.87"}, {"Year"="2013", "Airport"="Bologna Airport", "Country"="Italy", "Volume"="6193783", "Change"="3.95"}, {"Year"="2013", "Airport"="Bristol Airport", "Country"="United Kingdom", "Volume"="6131896", "Change"="3.55"}, {"Year"="2013", "Airport"="Faro Airport", "Country"="Portugal", "Volume"="5978685", "Change"="5.40"}, {"Year"="2013", "Airport"="EuroAirport Basel-Mulhouse-Freiburg", "Country"="Switzerland-France-Germany", "Volume"="5880771", "Change"="9.83"}, {"Year"="2013", "Airport"="Heraklion International Airport", "Country"="Greece", "Volume"="5792429", "Change"="15.52"}, {"Year"="2013", "Airport"="Ibiza Airport", "Country"="Spain", "Volume"="5726581", "Change"="3.09"}, {"Year"="2013", "Airport"="Naples Airport", "Country"="Italy", "Volume"="5444422", "Change"="-6.16"}, {"Year"="2013", "Airport"="Lanzarote Airport", "Country"="Spain", "Volume"="5334598", "Change"="3.21"}, {"Year"="2013", "Airport"="Langenhagen Airport", "Country"="Germany", "Volume"="5234909", "Change"="-1.00"}, {"Year"="2013", "Airport"="Gothenburg-Landvetter Airport", "Country"="Sweden", "Volume"="5004093", "Change"="3.07"}, {"Year"="2013", "Airport"="Larnaca International Airport", "Country"="Cyprus", "Volume"="4863577", "Change"="-5.86"}, {"Year"="2013", "Airport"="Riga International Airport", "Country"="Latvia", "Volume"="4793213", "Change"="0.53"}, {"Year"="2013", "Airport"="Rome Ciampino Airport", "Country"="Italy", "Volume"="4749251", "Change"="5.60"}, {"Year"="2013", "Airport"="Stavanger Sola Airport", "Country"="Norway", "Volume"="4668403", "Change"="5.76"}, {"Year"="2013", "Airport"="Valencia Airport", "Country"="Spain", "Volume"="4599990", "Change"="-3.20"}, {"Year"="2013", "Airport"="Bordeaux - Mérignac Airport", "Country"="France", "Volume"="4574357", "Change"="4.43"}, {"Year"="2013", "Airport"="Galileo Galilei Airport", "Country"="Italy", "Volume"="4479690", "Change"="-0.34"}, {"Year"="2013", "Airport"="Newcastle Airport", "Country"="United Kingdom", "Volume"="4420839", "Change"="1.25"}, {"Year"="2013", "Airport"="Palermo Airport", "Country"="Italy", "Volume"="4349672", "Change"="-5.62"}, {"Year"="2013", "Airport"="East Midlands Airport", "Country"="United Kingdom", "Volume"="4334117", "Change"="6.33"}, {"Year"="2013", "Airport"="Adana ?akirpa?a Airport", "Country"="Turkey", "Volume"="4316678", "Change"="14.28"}, {"Year"="2013", "Airport"="Trondheim Værnes Airport", "Country"="Norway", "Volume"="4311328", "Change"="3.63"}, {"Year"="2013", "Airport"="Koltsovo Airport", "Country"="Russia", "Volume"="4293002", "Change"="13.48"}, {"Year"="2013", "Airport"="Fuerteventura Airport", "Country"="Spain", "Volume"="4259341", "Change"="-3.18"}, {"Year"="2013", "Airport"="Rhodes International Airport", "Country"="Greece", "Volume"="4200068", "Change"="10.10"}, {"Year"="2013", "Airport"="Liverpool John Lennon Airport", "Country"="United Kingdom", "Volume"="4187493", "Change"="-6.18"}, {"Year"="2013", "Airport"="Thessaloniki International Airport, \"Macedonia\"", "Country"="Greece", "Volume"="4085032", "Change"="1.05"}, {"Year"="2013", "Airport"="Dalaman Airport", "Country"="Turkey", "Volume"="4057173", "Change"="6.49"}, {"Year"="2013", "Airport"="Malta International Airport", "Country"="Malta", "Volume"="4052000", "Change"="10.88"}, {"Year"="2013", "Airport"="Belfast International Airport", "Country"="United Kingdom", "Volume"="4023336", "Change"="-6.73"}, {"Year"="2013", "Airport"="Beauvais-Tillé Airport", "Country"="France", "Volume"="3952908", "Change"="2.34"}, {"Year"="2013", "Airport"="Nantes Atlantique Airport", "Country"="France", "Volume"="3930849", "Change"="8.24"}, {"Year"="2013", "Airport"="Bilbao Airport", "Country"="Spain", "Volume"="3800789", "Change"="-8.88"}, {"Year"="2013", "Airport"="Tolmachevo Airport", "Country"="Russia", "Volume"="3748211", "Change"="14.74"}, {"Year"="2013", "Airport"="San Pablo Airport", "Country"="Spain", "Volume"="3687727", "Change"="-14.08"}, {"Year"="2013", "Airport"="Kraków Airport", "Country"="Poland", "Volume"="3647616", "Change"="6.07"}, {"Year"="2012", "Airport"="London Heathrow Airport", "Country"="United Kingdom", "Volume"="70037417", "Change"="0.87"}, {"Year"="2012", "Airport"="Paris-Charles de Gaulle Airport", "Country"="France", "Volume"="61611934", "Change"="1.05"}, {"Year"="2012", "Airport"="Frankfurt Airport", "Country"="Germany", "Volume"="57520001", "Change"="1.92"}, {"Year"="2012", "Airport"="Amsterdam Airport Schiphol", "Country"="Netherlands", "Volume"="51035590", "Change"="2.57"}, {"Year"="2012", "Airport"="Madrid?Barajas Airport", "Country"="Spain", "Volume"="45190528", "Change"="-9.02"}, {"Year"="2012", "Airport"="Atatürk International Airport", "Country"="Turkey", "Volume"="45091962", "Change"="20.58"}, {"Year"="2012", "Airport"="Munich Airport", "Country"="Germany", "Volume"="38360604", "Change"="1.58"}, {"Year"="2012", "Airport"="Leonardo da Vinci-Fiumicino Airport", "Country"="Italy", "Volume"="36980911", "Change"="-1.78"}, {"Year"="2012", "Airport"="Barcelona El Prat Airport", "Country"="Spain", "Volume"="35144503", "Change"="2.17"}, {"Year"="2012", "Airport"="London Gatwick Airport", "Country"="United Kingdom", "Volume"="34235982", "Change"="1.67"}, {"Year"="2012", "Airport"="Domodedovo International Airport", "Country"="Russia", "Volume"="28165657", "Change"="9.59"}, {"Year"="2012", "Airport"="Paris-Orly Airport", "Country"="France", "Volume"="27232263", "Change"="0.34"}, {"Year"="2012", "Airport"="Sheremetyevo International Airport", "Country"="Russia", "Volume"="26032975", "Change"="16.47"}, {"Year"="2012", "Airport"="Antalya Airport", "Country"="Turkey", "Volume"="24993667", "Change"="-0.48"}, {"Year"="2012", "Airport"="Zürich Airport", "Country"="Switzerland", "Volume"="24802466", "Change"="1.91"}, {"Year"="2012", "Airport"="Copenhagen Airport, Kastrup", "Country"="Denmark", "Volume"="23336187", "Change"="2.69"}, {"Year"="2012", "Airport"="Palma de Mallorca Airport", "Country"="Spain", "Volume"="22666858", "Change"="-0.26"}, {"Year"="2012", "Airport"="Vienna International Airport", "Country"="Austria", "Volume"="22165794", "Change"="5.02"}, {"Year"="2012", "Airport"="Oslo Gardermoen International Airport", "Country"="Norway", "Volume"="22080433", "Change"="4.63"}, {"Year"="2012", "Airport"="Düsseldorf International Airport", "Country"="Germany", "Volume"="20833246", "Change"="2.43"}, {"Year"="2012", "Airport"="Manchester Airport", "Country"="United Kingdom", "Volume"="19736502", "Change"="4.47"}, {"Year"="2012", "Airport"="Stockholm-Arlanda Airport", "Country"="Sweden", "Volume"="19642029", "Change"="3.00"}, {"Year"="2012", "Airport"="Dublin Airport", "Country"="Ireland", "Volume"="19099649", "Change"="1.91"}, {"Year"="2012", "Airport"="Brussels Airport", "Country"="Belgium", "Volume"="18971332", "Change"="0.99"}, {"Year"="2012", "Airport"="Malpensa Airport", "Country"="Italy", "Volume"="18537301", "Change"="-3.97"}, {"Year"="2012", "Airport"="Berlin Tegel Airport", "Country"="Germany", "Volume"="18164203", "Change"="7.35"}, {"Year"="2012", "Airport"="London Stansted Airport", "Country"="United Kingdom", "Volume"="17472699", "Change"="-3.21"}, {"Year"="2012", "Airport"="Lisbon Portela Airport", "Country"="Portugal", "Volume"="15301176", "Change"="3.35"}, {"Year"="2012", "Airport"="Helsinki Airport", "Country"="Finland", "Volume"="14858215", "Change"="-0.05"}, {"Year"="2012", "Airport"="Sabiha Gökçen Airport", "Country"="Turkey", "Volume"="14487242", "Change"="13.63"}, {"Year"="2012", "Airport"="Geneva International Airport", "Country"="Switzerland", "Volume"="13899422", "Change"="6.01"}, {"Year"="2012", "Airport"="Hamburg Airport", "Country"="Germany", "Volume"="13697402", "Change"="1.03"}, {"Year"="2012", "Airport"="Athens International Airport", "Country"="Greece", "Volume"="12944041", "Change"="-10.40"}, {"Year"="2012", "Airport"="Málaga Airport", "Country"="Spain", "Volume"="12581944", "Change"="-1.88"}, {"Year"="2012", "Airport"="Nice Côte d'Azur Airport", "Country"="France", "Volume"="11189896", "Change"="7.37"}, {"Year"="2012", "Airport"="Pulkovo Airport", "Country"="Russia", "Volume"="11154560", "Change"="16.06"}, {"Year"="2012", "Airport"="Václav Havel Airport Prague", "Country"="Czech Republic", "Volume"="10807890", "Change"="-8.32"}, {"Year"="2012", "Airport"="Gran Canaria Airport", "Country"="Spain", "Volume"="9892067", "Change"="-6.14"}, {"Year"="2012", "Airport"="Stuttgart Airport", "Country"="Germany", "Volume"="9720877", "Change"="1.45"}, {"Year"="2012", "Airport"="Vnukovo International Airport", "Country"="Russia", "Volume"="9690000", "Change"="18.21"}, {"Year"="2012", "Airport"="London Luton Airport", "Country"="United Kingdom", "Volume"="9617697", "Change"="1.09"}, {"Year"="2012", "Airport"="Frederic Chopin Airport", "Country"="Poland", "Volume"="9587842", "Change"="2.68"}, {"Year"="2012", "Airport"="Adnan Menderes Airport", "Country"="Turkey", "Volume"="9356284", "Change"="9.77"}, {"Year"="2012", "Airport"="Cologne Bonn Airport", "Country"="Germany", "Volume"="9280070", "Change"="-3.57"}, {"Year"="2012", "Airport"="Esenbo?a Airport", "Country"="Turkey", "Volume"="9237886", "Change"="8.87"}, {"Year"="2012", "Airport"="Linate Airport", "Country"="Italy", "Volume"="9229890", "Change"="1.11"}, {"Year"="2012", "Airport"="Edinburgh Airport", "Country"="United Kingdom", "Volume"="9195061", "Change"="-2.03"}, {"Year"="2012", "Airport"="Birmingham Airport", "Country"="United Kingdom", "Volume"="8922539", "Change"="3.55"}, {"Year"="2012", "Airport"="Orio al Serio Airport", "Country"="Italy", "Volume"="8890720", "Change"="5.59"}, {"Year"="2012", "Airport"="Alicante Airport", "Country"="Spain", "Volume"="8855444", "Change"="-10.67"}, {"Year"="2012", "Airport"="Tenerife South Airport", "Country"="Spain", "Volume"="8530729", "Change"="-1.45"}, {"Year"="2012", "Airport"="Budapest Liszt Ferenc International Airport", "Country"="Hungary", "Volume"="8504020", "Change"="-4.67"}, {"Year"="2012", "Airport"="Boryspil International Airport", "Country"="Ukraine", "Volume"="8478091", "Change"="5.36"}, {"Year"="2012", "Airport"="Lyon-Saint Exupéry Airport", "Country"="France", "Volume"="8451039", "Change"="0.16"}, {"Year"="2012", "Airport"="Marseille Provence Airport", "Country"="France", "Volume"="8295479", "Change"="12.61"}, {"Year"="2012", "Airport"="Venice Marco Polo Airport", "Country"="Italy", "Volume"="8188455", "Change"="-4.62"}, {"Year"="2012", "Airport"="Blagnac Airport", "Country"="France", "Volume"="7559350", "Change"="8.17"}, {"Year"="2012", "Airport"="Glasgow International Airport", "Country"="United Kingdom", "Volume"="7157859", "Change"="4.04"}, {"Year"="2012", "Airport"="Henri Coand? International Airport", "Country"="Romania", "Volume"="7120067", "Change"="41.01"}, {"Year"="2012", "Airport"="Berlin Schönefeld Airport", "Country"="Germany", "Volume"="7097274", "Change"="-0.23"}, {"Year"="2012", "Airport"="Brussels South Charleroi Airport", "Country"="Belgium", "Volume"="6516427", "Change"="10.43"}, {"Year"="2012", "Airport"="Catania-Fontanarossa Airport", "Country"="Italy", "Volume"="6246888", "Change"="-8.05"}, {"Year"="2012", "Airport"="Francisco de Sá Carneiro Airport", "Country"="Portugal", "Volume"="6050094", "Change"="0.76"}, {"Year"="2012", "Airport"="Bologna Airport", "Country"="Italy", "Volume"="5958648", "Change"="1.24"}, {"Year"="2012", "Airport"="Bristol Airport", "Country"="United Kingdom", "Volume"="5921530", "Change"="2.44"}, {"Year"="2012", "Airport"="Bergen Flesland Airport", "Country"="Norway", "Volume"="5814413", "Change"="3.80"}, {"Year"="2012", "Airport"="Naples Airport", "Country"="Italy", "Volume"="5801836", "Change"="0.57"}, {"Year"="2012", "Airport"="Faro Airport", "Country"="Portugal", "Volume"="5672377", "Change"="1.01"}, {"Year"="2012", "Airport"="Ibiza Airport", "Country"="Spain", "Volume"="5555048", "Change"="-1.56"}, {"Year"="2012", "Airport"="EuroAirport Basel-Mulhouse-Freiburg", "Country"="Switzerland-France-Germany", "Volume"="5354674", "Change"="5.96"}, {"Year"="2012", "Airport"="Langenhagen Airport", "Country"="Germany", "Volume"="5287831", "Change"="-0.98"}, {"Year"="2012", "Airport"="Lanzarote Airport", "Country"="Spain", "Volume"="5168775", "Change"="-6.76"}, {"Year"="2012", "Airport"="Larnaca International Airport", "Country"="Cyprus", "Volume"="5166224", "Change"="-6.20"}, {"Year"="2012", "Airport"="Heraklion International Airport", "Country"="Greece", "Volume"="5014312", "Change"="-5.26"}, {"Year"="2012", "Airport"="Gothenburg-Landvetter Airport", "Country"="Sweden", "Volume"="4854888", "Change"="-1.05"}, {"Year"="2012", "Airport"="Riga International Airport", "Country"="Latvia", "Volume"="4767878", "Change"="-6.64"}, {"Year"="2012", "Airport"="Valencia Airport", "Country"="Spain", "Volume"="4752020", "Change"="-4.57"}, {"Year"="2012", "Airport"="Palermo Airport", "Country"="Italy", "Volume"="4608533", "Change"="-7.70"}, {"Year"="2012", "Airport"="Rome Ciampino Airport", "Country"="Italy", "Volume"="4497376", "Change"="-5.95"}, {"Year"="2012", "Airport"="Galileo Galilei Airport", "Country"="Italy", "Volume"="4494915", "Change"="-0.70"}, {"Year"="2012", "Airport"="Liverpool John Lennon Airport", "Country"="United Kingdom", "Volume"="4463257", "Change"="-15.00"}, {"Year"="2012", "Airport"="Stavanger Sola Airport", "Country"="Norway", "Volume"="4413987", "Change"="6.83"}, {"Year"="2012", "Airport"="Fuerteventura Airport", "Country"="Spain", "Volume"="4399023", "Change"="-11.10"}, {"Year"="2012", "Airport"="Bordeaux - Mérignac Airport", "Country"="France", "Volume"="4380145", "Change"="6.38"}, {"Year"="2012", "Airport"="Newcastle Airport", "Country"="United Kingdom", "Volume"="4366196", "Change"="0.46"}, {"Year"="2012", "Airport"="Belfast International Airport", "Country"="United Kingdom", "Volume"="4313685", "Change"="5.12"}, {"Year"="2012", "Airport"="San Pablo Airport", "Country"="Spain", "Volume"="4292020", "Change"="-13.46"}, {"Year"="2012", "Airport"="Bilbao Airport", "Country"="Spain", "Volume"="4171065", "Change"="3.09"}, {"Year"="2012", "Airport"="Trondheim Værnes Airport", "Country"="Norway", "Volume"="4160162", "Change"="5.95"}, {"Year"="2012", "Airport"="East Midlands Airport", "Country"="United Kingdom", "Volume"="4076178", "Change"="-3.30"}, {"Year"="2012", "Airport"="Thessaloniki International Airport, \"Macedonia\"", "Country"="Greece", "Volume"="4042539", "Change"="-0.47"}, {"Year"="2012", "Airport"="Beauvais-Tillé Airport", "Country"="France", "Volume"="3862431", "Change"="5.02"}, {"Year"="2012", "Airport"="Rhodes International Airport", "Country"="Greece", "Volume"="3814706", "Change"="-8.06"}, {"Year"="2012", "Airport"="Dalaman Airport", "Country"="Turkey", "Volume"="3810015", "Change"="2.06"}, {"Year"="2012", "Airport"="Koltsovo Airport", "Country"="Russia", "Volume"="3783069", "Change"="12.73"}, {"Year"="2012", "Airport"="Bari Airport", "Country"="Italy", "Volume"="3780112", "Change"="1.46"}, {"Year"="2012", "Airport"="Adana ?akirpa?a Airport", "Country"="Turkey", "Volume"="3777348", "Change"="16.55"}, {"Year"="2012", "Airport"="Los Rodeos Airport", "Country"="Spain", "Volume"="3717944", "Change"="-9.21"}, {"Year"="2012", "Airport"="Malta International Airport", "Country"="Malta", "Volume"="3654283", "Change"="4.10"}, {"Year"="2012", "Airport"="Nantes Atlantique Airport", "Country"="France", "Volume"="3631693", "Change"="11.88"}, {"Year"="2011", "Airport"="London Heathrow Airport", "Country"="United Kingdom", "Volume"="69433230", "Change"="5.39"}, {"Year"="2011", "Airport"="Paris-Charles de Gaulle Airport", "Country"="France", "Volume"="60970551", "Change"="4.82"}, {"Year"="2011", "Airport"="Frankfurt Airport", "Country"="Germany", "Volume"="56436255", "Change"="6.46"}, {"Year"="2011", "Airport"="Amsterdam Airport Schiphol", "Country"="Netherlands", "Volume"="49755252", "Change"="10.05"}, {"Year"="2011", "Airport"="Madrid Barajas Airport", "Country"="Spain", "Volume"="49671270", "Change"="-0.39"}, {"Year"="2011", "Airport"="Munich Airport", "Country"="Germany", "Volume"="37763701", "Change"="8.76"}, {"Year"="2011", "Airport"="Rome-Fiumicino Airport", "Country"="Italy", "Volume"="37651700", "Change"="3.62"}, {"Year"="2011", "Airport"="Atatürk International Airport", "Country"="Turkey", "Volume"="37394694", "Change"="16.34"}, {"Year"="2011", "Airport"="Barcelona El Prat Airport", "Country"="Spain", "Volume"="34398226", "Change"="17.76"}, {"Year"="2011", "Airport"="London Gatwick Airport", "Country"="United Kingdom", "Volume"="33674264", "Change"="7.33"}, {"Year"="2011", "Airport"="Paris-Orly Airport", "Country"="France", "Volume"="27139076", "Change"="7.68"}, {"Year"="2011", "Airport"="Domodedovo International Airport", "Country"="Russia", "Volume"="25701610", "Change"="15.49"}, {"Year"="2011", "Airport"="Antalya Airport", "Country"="Turkey", "Volume"="25113635", "Change"="14.09"}, {"Year"="2011", "Airport"="Zurich Airport", "Country"="Switzerland", "Volume"="24337954", "Change"="6.38"}, {"Year"="2011", "Airport"="Palma de Mallorca Airport", "Country"="Spain", "Volume"="22726707", "Change"="7.62"}, {"Year"="2011", "Airport"="Copenhagen Airport", "Country"="Denmark", "Volume"="22725517", "Change"="5.69"}, {"Year"="2011", "Airport"="Sheremetyevo International Airport", "Country"="Russia", "Volume"="22351317", "Change"="16.88"}, {"Year"="2011", "Airport"="Vienna International Airport", "Country"="Austria", "Volume"="21106292", "Change"="7.19"}, {"Year"="2011", "Airport"="Oslo-Gardermoen Airport", "Country"="Norway", "Volume"="21103623", "Change"="10.54"}, {"Year"="2011", "Airport"="Düsseldorf International Airport", "Country"="Germany", "Volume"="20339466", "Change"="7.12"}, {"Year"="2011", "Airport"="Milan Malpensa Airport", "Country"="Italy", "Volume"="19303131", "Change"="1.88"}, {"Year"="2011", "Airport"="Stockholm-Arlanda Airport", "Country"="Sweden", "Volume"="19069065", "Change"="12.42"}, {"Year"="2011", "Airport"="Manchester Airport", "Country"="United Kingdom", "Volume"="18892756", "Change"="6.38"}, {"Year"="2011", "Airport"="Brussels Airport", "Country"="Belgium", "Volume"="18786034", "Change"="9.34"}, {"Year"="2011", "Airport"="Dublin Airport", "Country"="Ireland", "Volume"="18740593", "Change"="1.68"}, {"Year"="2011", "Airport"="London Stansted Airport", "Country"="United Kingdom", "Volume"="18052843", "Change"="-2.80"}, {"Year"="2011", "Airport"="Berlin Tegel Airport", "Country"="Germany", "Volume"="16919820", "Change"="12.61"}, {"Year"="2011", "Airport"="Helsinki Airport", "Country"="Finland", "Volume"="14865871", "Change"="15.39"}, {"Year"="2011", "Airport"="Lisbon Portela Airport", "Country"="Portugal", "Volume"="14805624", "Change"="5.49"}, {"Year"="2011", "Airport"="Athens International Airport", "Country"="Greece", "Volume"="14446963", "Change"="-5.59"}, {"Year"="2011", "Airport"="Hamburg Airport", "Country"="Germany", "Volume"="13558261", "Change"="4.60"}, {"Year"="2011", "Airport"="Geneva Cointrin International Airport", "Country"="Switzerland", "Volume"="13111741", "Change"="11.25"}, {"Year"="2011", "Airport"="Málaga Airport", "Country"="Spain", "Volume"="12823117", "Change"="6.29"}, {"Year"="2011", "Airport"="Sabiha Gökçen Airport", "Country"="Turkey", "Volume"="12749230", "Change"="13.94"}, {"Year"="2011", "Airport"="Václav Havel Airport Prague", "Country"="Czech Republic", "Volume"="11788629", "Change"="2.01"}, {"Year"="2011", "Airport"="Gran Canaria Airport", "Country"="Spain", "Volume"="10538829", "Change"="11.10"}, {"Year"="2011", "Airport"="Nice Côte d'Azur Airport", "Country"="France", "Volume"="10422073", "Change"="8.53"}, {"Year"="2011", "Airport"="Alicante Airport", "Country"="Spain", "Volume"="9913731", "Change"="5.66"}, {"Year"="2011", "Airport"="Cologne Bonn Airport", "Country"="Germany", "Volume"="9623398", "Change"="-2.30"}, {"Year"="2011", "Airport"="Pulkovo Airport", "Country"="Russia", "Volume"="9610767", "Change"="14.53"}, {"Year"="2011", "Airport"="Stuttgart Airport", "Country"="Germany", "Volume"="9582265", "Change"="3.95"}, {"Year"="2011", "Airport"="London Luton Airport", "Country"="United Kingdom", "Volume"="9513704", "Change"="8.87"}, {"Year"="2011", "Airport"="Edinburgh Airport", "Country"="United Kingdom", "Volume"="9385245", "Change"="9.17"}, {"Year"="2011", "Airport"="Frederic Chopin Airport", "Country"="Poland", "Volume"="9337734", "Change"="7.18"}, {"Year"="2011", "Airport"="Milan Linate Airport", "Country"="Italy", "Volume"="9128522", "Change"="10.03"}, {"Year"="2011", "Airport"="Budapest Liszt Ferenc International Airport", "Country"="Hungary", "Volume"="8920653", "Change"="8.92"}, {"Year"="2011", "Airport"="Tenerife South Airport", "Country"="Spain", "Volume"="8656487", "Change"="17.63"}, {"Year"="2011", "Airport"="Birmingham Airport", "Country"="United Kingdom", "Volume"="8616296", "Change"="0.51"}, {"Year"="2011", "Airport"="Venice Marco Polo Airport", "Country"="Italy", "Volume"="8584651", "Change"="25.24"}, {"Year"="2011", "Airport"="Adnan Menderes Airport", "Country"="Turkey", "Volume"="8523533", "Change"="13.87"}, {"Year"="2011", "Airport"="Esenbo?a Airport", "Country"="Turkey", "Volume"="8485467", "Change"="9.29"}, {"Year"="2011", "Airport"="Lyon-Saint Exupéry Airport", "Country"="France", "Volume"="8437141", "Change"="5.74"}, {"Year"="2011", "Airport"="Bergamo Orio al Serio airport", "Country"="Italy", "Volume"="8419948", "Change"="9.67"}, {"Year"="2011", "Airport"="Vnukovo International Airport", "Country"="Russia", "Volume"="8197162", "Change"="-13.35"}, {"Year"="2011", "Airport"="Boryspil International Airport", "Country"="Ukraine", "Volume"="8047115", "Change"="20.24"}, {"Year"="2011", "Airport"="Marseille Provence Airport", "Country"="France", "Volume"="7366873", "Change"="-2.10"}, {"Year"="2011", "Airport"="Berlin Schönefeld Airport", "Country"="Germany", "Volume"="7113989", "Change"="-2.52"}, {"Year"="2011", "Airport"="Blagnac Airport", "Country"="France", "Volume"="6988140", "Change"="9.09"}, {"Year"="2011", "Airport"="Glasgow International Airport", "Country"="United Kingdom", "Volume"="6880217", "Change"="5.06"}, {"Year"="2011", "Airport"="Catania-Fontanarossa Airport", "Country"="Italy", "Volume"="6794063", "Change"="7.53"}, {"Year"="2011", "Airport"="Francisco de Sá Carneiro Airport", "Country"="Portugal", "Volume"="6004589", "Change"="13.74"}, {"Year"="2011", "Airport"="Brussels South Charleroi Airport", "Country"="Belgium", "Volume"="5901007", "Change"="13.58"}, {"Year"="2011", "Airport"="Bologna Airport", "Country"="Italy", "Volume"="5885884", "Change"="6.96"}, {"Year"="2011", "Airport"="Bristol Airport", "Country"="United Kingdom", "Volume"="5780746", "Change"="0.58"}, {"Year"="2011", "Airport"="Naples Airport", "Country"="Italy", "Volume"="5768873", "Change"="3.54"}, {"Year"="2011", "Airport"="Ibiza Airport", "Country"="Spain", "Volume"="5643180", "Change"="11.95"}, {"Year"="2011", "Airport"="Faro Airport", "Country"="Portugal", "Volume"="5615580", "Change"="5.24"}, {"Year"="2011", "Airport"="Bergen Airport", "Country"="Norway", "Volume"="5814413", "Change"="14.50"}, {"Year"="2011", "Airport"="Lanzarote Airport", "Country"="Spain", "Volume"="5543744", "Change"="12.26"}, {"Year"="2011", "Airport"="Larnaca International Airport", "Country"="Cyprus", "Volume"="5507762", "Change"="2.61"}, {"Year"="2011", "Airport"="Langenhagen Airport", "Country"="Germany", "Volume"="5340264", "Change"="5.54"}, {"Year"="2011", "Airport"="Heraklion International Airport", "Country"="Greece", "Volume"="5292687", "Change"="7.85"}, {"Year"="2011", "Airport"="Liverpool John Lennon Airport", "Country"="United Kingdom", "Volume"="5251161", "Change"="4.73"}, {"Year"="2011", "Airport"="Riga International Airport", "Country"="Latvia", "Volume"="5106926", "Change"="9.50"}, {"Year"="2011", "Airport"="EuroAirport Basel-Mulhouse-Freiburg", "Country"="Switzerland-France-Germany", "Volume"="5053664", "Change"="22.39"}, {"Year"="2011", "Airport"="Henri Coand? International Airport", "Country"="Romania", "Volume"="5049443", "Change"="2.67"}, {"Year"="2011", "Airport"="Palermo Airport", "Country"="Italy", "Volume"="4992798", "Change"="14.96"}, {"Year"="2011", "Airport"="Valencia Airport", "Country"="Spain", "Volume"="4979511", "Change"="0.92"}, {"Year"="2011", "Airport"="San Pablo Airport", "Country"="Spain", "Volume"="4959359", "Change"="17.39"}, {"Year"="2011", "Airport"="Fuerteventura Airport", "Country"="Spain", "Volume"="4948018", "Change"="18.56"}, {"Year"="2011", "Airport"="Gothenburg-Landvetter Airport", "Country"="Sweden", "Volume"="4906639", "Change"="18.71"}, {"Year"="2011", "Airport"="Rome Ciampino Airport", "Country"="Italy", "Volume"="4781731", "Change"="5.51"}, {"Year"="2011", "Airport"="Pisa Airport", "Country"="Italy", "Volume"="4526723", "Change"="11.52"}, {"Year"="2011", "Airport"="Newcastle Airport", "Country"="United Kingdom", "Volume"="4346270", "Change"="-0.23"}, {"Year"="2011", "Airport"="East Midlands Airport", "Country"="United Kingdom", "Volume"="4215192", "Change"="2.47"}, {"Year"="2011", "Airport"="Rhodes International Airport", "Country"="Greece", "Volume"="4149274", "Change"="15.69"}, {"Year"="2011", "Airport"="Stavanger Airport", "Country"="Norway", "Volume"="4131974", "Change"="12.44"}, {"Year"="2011", "Airport"="Bordeaux - Mérignac Airport", "Country"="France", "Volume"="4117303", "Change"="12.38"}, {"Year"="2011", "Airport"="Belfast International Airport", "Country"="United Kingdom", "Volume"="4103620", "Change"="2.18"}, {"Year"="2011", "Airport"="Los Rodeos Airport", "Country"="Spain", "Volume"="4095103", "Change"="1.08"}, {"Year"="2011", "Airport"="Thessaloniki International Airport, \"Macedonia\"", "Country"="Greece", "Volume"="4061697", "Change"="3.86"}, {"Year"="2011", "Airport"="Bilbao Airport", "Country"="Spain", "Volume"="4046172", "Change"="4.04"}, {"Year"="2011", "Airport"="Nuremberg Airport", "Country"="Germany", "Volume"="3962617", "Change"="-2.61"}, {"Year"="2011", "Airport"="Trondheim Airport", "Country"="Norway", "Volume"="3926461", "Change"="11.49"}, {"Year"="2011", "Airport"="Dalaman Airport", "Country"="Turkey", "Volume"="3732941", "Change"="-1.40"}, {"Year"="2011", "Airport"="Bari Airport", "Country"="Italy", "Volume"="3725629", "Change"="9.64"}, {"Year"="2011", "Airport"="Turin Airport", "Country"="Italy", "Volume"="3710485", "Change"="4.45"}, {"Year"="2011", "Airport"="Cagliari-Elmas Airport", "Country"="Italy", "Volume"="3698982", "Change"="7.43"}, {"Year"="2011", "Airport"="Beauvais-Tillé Airport", "Country"="France", "Volume"="3677825", "Change"="25.45"}, {"Year"="2011", "Airport"="Malta International Airport", "Country"="Malta", "Volume"="3510213", "Change"="6.36"}, {"Year"="2010", "Airport"="London Heathrow Airport", "Country"="United Kingdom", "Volume"="65881660", "Change"="-0.24"}, {"Year"="2010", "Airport"="Paris-Charles de Gaulle Airport", "Country"="France", "Volume"="58164612", "Change"="0.45"}, {"Year"="2010", "Airport"="Frankfurt Airport", "Country"="Germany", "Volume"="53009221", "Change"="4.08"}, {"Year"="2010", "Airport"="Barajas Airport", "Country"="Spain", "Volume"="49866113", "Change"="2.95"}, {"Year"="2010", "Airport"="Amsterdam Airport Schiphol", "Country"="Netherlands", "Volume"="45211749", "Change"="3.77"}, {"Year"="2010", "Airport"="Leonardo da Vinci-Fiumicino Airport", "Country"="Italy", "Volume"="36337050", "Change"="7.48"}, {"Year"="2010", "Airport"="Munich Airport", "Country"="Germany", "Volume"="34721605", "Change"="6.24"}, {"Year"="2010", "Airport"="Atatürk International Airport", "Country"="Turkey", "Volume"="32143819", "Change"="7.82"}, {"Year"="2010", "Airport"="Gatwick Airport", "Country"="United Kingdom", "Volume"="31375290", "Change"="-3.14"}, {"Year"="2010", "Airport"="Barcelona El Prat Airport", "Country"="Spain", "Volume"="29209536", "Change"="6.52"}, {"Year"="2010", "Airport"="Paris-Orly Airport", "Country"="France", "Volume"="25203969", "Change"="0.38"}, {"Year"="2010", "Airport"="Zurich Airport", "Country"="Switzerland", "Volume"="22878251", "Change"="4.34"}, {"Year"="2010", "Airport"="Domodedovo International Airport", "Country"="Russia", "Volume"="22253529", "Change"="19.16"}, {"Year"="2010", "Airport"="Antalya Airport", "Country"="Turkey", "Volume"="22013027", "Change"="19.99"}, {"Year"="2010", "Airport"="Copenhagen Airport", "Country"="Denmark", "Volume"="21501750", "Change"="9.06"}, {"Year"="2010", "Airport"="Palma de Mallorca Airport", "Country"="Spain", "Volume"="21117417", "Change"="-0.40"}, {"Year"="2010", "Airport"="Vienna International Airport", "Country"="Austria", "Volume"="19691206", "Change"="8.71"}, {"Year"="2010", "Airport"="Sheremetyevo International Airport", "Country"="Russia", "Volume"="19123007", "Change"="29.52"}, {"Year"="2010", "Airport"="Oslo-Gardermoen Airport", "Country"="Norway", "Volume"="19091036", "Change"="5.55"}, {"Year"="2010", "Airport"="Düsseldorf International Airport", "Country"="Germany", "Volume"="18988149", "Change"="6.71"}, {"Year"="2010", "Airport"="Malpensa Airport", "Country"="Italy", "Volume"="18947808", "Change"="7.95"}, {"Year"="2010", "Airport"="London Stansted Airport", "Country"="United Kingdom", "Volume"="18573592", "Change"="-6.93"}, {"Year"="2010", "Airport"="Dublin Airport", "Country"="Ireland", "Volume"="18431064", "Change"="-10.11"}, {"Year"="2010", "Airport"="Manchester Airport", "Country"="United Kingdom", "Volume"="17759173", "Change"="-5.16"}, {"Year"="2010", "Airport"="Brussels Airport", "Country"="Belgium", "Volume"="17180606", "Change"="1.07"}, {"Year"="2010", "Airport"="Stockholm-Arlanda Airport", "Country"="Sweden", "Volume"="16962416", "Change"="5.59"}, {"Year"="2010", "Airport"="Athens International Airport", "Country"="Greece", "Volume"="15303127", "Change"="-5.69"}, {"Year"="2010", "Airport"="Berlin Tegel Airport", "Country"="Germany", "Volume"="15025600", "Change"="5.96"}, {"Year"="2010", "Airport"="Lisbon Portela Airport", "Country"="Portugal", "Volume"="14035273", "Change"="5.70"}, {"Year"="2010", "Airport"="Hamburg Airport", "Country"="Germany", "Volume"="12962429", "Change"="5.99"}, {"Year"="2010", "Airport"="Helsinki Airport", "Country"="Finland", "Volume"="12883399", "Change"="2.32"}, {"Year"="2010", "Airport"="Málaga Airport", "Country"="Spain", "Volume"="12064521", "Change"="3.80"}, {"Year"="2010", "Airport"="Geneva Cointrin International Airport", "Country"="Switzerland", "Volume"="11785522", "Change"="4.07"}, {"Year"="2010", "Airport"="Ruzyn? Airport", "Country"="Czech Republic", "Volume"="11556858", "Change"="-0.74"}, {"Year"="2010", "Airport"="Sabiha Gökçen Airport", "Country"="Turkey", "Volume"="11189678", "Change"="68.51"}, {"Year"="2010", "Airport"="Cologne Bonn Airport", "Country"="Germany", "Volume"="9849779", "Change"="1.13"}, {"Year"="2010", "Airport"="Nice Côte d'Azur Airport", "Country"="France", "Volume"="9603014", "Change"="-2.32"}, {"Year"="2010", "Airport"="Gran Canaria Airport", "Country"="Spain", "Volume"="9486035", "Change"="3.61"}, {"Year"="2010", "Airport"="Vnukovo International Airport", "Country"="Russia", "Volume"="9460292", "Change"="22.37"}, {"Year"="2010", "Airport"="Alicante Airport", "Country"="Spain", "Volume"="9382931", "Change"="2.66"}, {"Year"="2010", "Airport"="Stuttgart Airport", "Country"="Germany", "Volume"="9218095", "Change"="3.17"}, {"Year"="2010", "Airport"="London Luton Airport", "Country"="United Kingdom", "Volume"="8738712", "Change"="-4.19"}, {"Year"="2010", "Airport"="Frederic Chopin Airport", "Country"="Poland", "Volume"="8712384", "Change"="4.70"}, {"Year"="2010", "Airport"="Edinburgh Airport", "Country"="United Kingdom", "Volume"="8596715", "Change"="-5.00"}, {"Year"="2010", "Airport"="Birmingham Airport", "Country"="United Kingdom", "Volume"="8572398", "Change"="-5.83"}, {"Year"="2010", "Airport"="Pulkovo Airport", "Country"="Russia", "Volume"="8391281", "Change"="24.17"}, {"Year"="2010", "Airport"="Linate Airport", "Country"="Italy", "Volume"="8296450", "Change"="0.02"}, {"Year"="2010", "Airport"="Budapest Liszt Ferenc International Airport", "Country"="Hungary", "Volume"="8190089", "Change"="1.17"}, {"Year"="2010", "Airport"="Lyon-Saint Exupéry Airport", "Country"="France", "Volume"="7979228", "Change"="3.39"}, {"Year"="2010", "Airport"="Esenbo?a Airport", "Country"="Turkey", "Volume"="7763914", "Change"="27.60"}, {"Year"="2010", "Airport"="Orio al Serio Airport", "Country"="Italy", "Volume"="7677224", "Change"="7.26"}, {"Year"="2010", "Airport"="Marseille Provence Airport", "Country"="France", "Volume"="7524886", "Change"="3.22"}, {"Year"="2010", "Airport"="Adnan Menderes Airport", "Country"="Turkey", "Volume"="7485098", "Change"="20.69"}, {"Year"="2010", "Airport"="Tenerife South Airport", "Country"="Spain", "Volume"="7358986", "Change"="3.53"}, {"Year"="2010", "Airport"="Berlin Schönefeld Airport", "Country"="Germany", "Volume"="7297911", "Change"="7.37"}, {"Year"="2010", "Airport"="Venice Marco Polo Airport", "Country"="Italy", "Volume"="6854595", "Change"="2.28"}, {"Year"="2010", "Airport"="Boryspil International Airport", "Country"="Ukraine", "Volume"="6692382", "Change"="15.49"}, {"Year"="2010", "Airport"="Glasgow International Airport", "Country"="United Kingdom", "Volume"="6548865", "Change"="-9.36"}, {"Year"="2010", "Airport"="Blagnac Airport", "Country"="France", "Volume"="6405906", "Change"="2.04"}, {"Year"="2010", "Airport"="Catania-Fontanarossa Airport", "Country"="Italy", "Volume"="6318177", "Change"="6.52"}, {"Year"="2010", "Airport"="Bristol Airport", "Country"="United Kingdom", "Volume"="5747604", "Change"="1.86"}, {"Year"="2010", "Airport"="Naples Airport", "Country"="Italy", "Volume"="5571738", "Change"="4.91"}, {"Year"="2010", "Airport"="Bologna Airport", "Country"="Italy", "Volume"="5503106", "Change"="15.26"}, {"Year"="2010", "Airport"="Larnaca International Airport", "Country"="Cyprus", "Volume"="5367724", "Change"="3.85"}, {"Year"="2010", "Airport"="Faro Airport", "Country"="Portugal", "Volume"="5336173", "Change"="5.31"}, {"Year"="2010", "Airport"="Francisco de Sá Carneiro Airport", "Country"="Portugal", "Volume"="5279362", "Change"="17.08"}, {"Year"="2010", "Airport"="Brussels South Charleroi Airport", "Country"="Belgium", "Volume"="5195372", "Change"="31.96"}, {"Year"="2010", "Airport"="Bergen Airport", "Country"="Norway", "Volume"="5078267", "Change"="4.43"}, {"Year"="2010", "Airport"="Langenhagen Airport", "Country"="Germany", "Volume"="5059800", "Change"="1.81"}, {"Year"="2010", "Airport"="Ibiza Airport", "Country"="Spain", "Volume"="5040800", "Change"="10.23"}, {"Year"="2010", "Airport"="Liverpool John Lennon Airport", "Country"="United Kingdom", "Volume"="5013940", "Change"="2.65"}, {"Year"="2010", "Airport"="Lanzarote Airport", "Country"="Spain", "Volume"="4938343", "Change"="5.03"}, {"Year"="2010", "Airport"="Valencia Airport", "Country"="Spain", "Volume"="4934268", "Change"="3.90"}, {"Year"="2010", "Airport"="Henri Coand? International Airport", "Country"="Romania", "Volume"="4917952", "Change"="9.69"}, {"Year"="2010", "Airport"="Heraklion International Airport", "Country"="Greece", "Volume"="4907337", "Change"="-2.88"}, {"Year"="2010", "Airport"="Girona-Costa Brava Airport", "Country"="Spain", "Volume"="4863954", "Change"="-8.00"}, {"Year"="2010", "Airport"="Riga International Airport", "Country"="Latvia", "Volume"="4663647", "Change"="14.67"}, {"Year"="2010", "Airport"="Rome Ciampino Airport", "Country"="Italy", "Volume"="4531834", "Change"="-4.75"}, {"Year"="2010", "Airport"="Newcastle Airport", "Country"="United Kingdom", "Volume"="4356130", "Change"="-5.05"}, {"Year"="2010", "Airport"="Palermo Airport", "Country"="Italy", "Volume"="4343227", "Change"="-0.17"}, {"Year"="2010", "Airport"="San Pablo Airport", "Country"="Spain", "Volume"="4224718", "Change"="4.28"}, {"Year"="2010", "Airport"="Fuerteventura Airport", "Country"="Spain", "Volume"="4173590", "Change"="11.64"}, {"Year"="2010", "Airport"="Gothenburg-Landvetter Airport", "Country"="Sweden", "Volume"="4133299", "Change"="12.04"}, {"Year"="2010", "Airport"="EuroAirport Basel-Mulhouse-Freiburg", "Country"="Switzerland-France-Germany", "Volume"="4129186", "Change"="7.24"}, {"Year"="2010", "Airport"="East Midlands Airport", "Country"="United Kingdom", "Volume"="4113501", "Change"="-11.69"}, {"Year"="2010", "Airport"="Nuremberg Airport", "Country"="Germany", "Volume"="4068799", "Change"="2.60"}, {"Year"="2010", "Airport"="Galileo Galilei Airport", "Country"="Italy", "Volume"="4058957", "Change"="1.18"}, {"Year"="2010", "Airport"="Los Rodeos Airport", "Country"="Spain", "Volume"="4051356", "Change"="-0.07"}, {"Year"="2010", "Airport"="Belfast International Airport", "Country"="United Kingdom", "Volume"="4016170", "Change"="-11.66"}, {"Year"="2010", "Airport"="Thessaloniki International Airport, \"Macedonia\"", "Country"="Greece", "Volume"="3910751", "Change"="-4.71"}, {"Year"="2010", "Airport"="Bilbao Airport", "Country"="Spain", "Volume"="3888955", "Change"="6.40"}, {"Year"="2010", "Airport"="Dalaman Airport", "Country"="Turkey", "Volume"="3785779", "Change"="5.22"}, {"Year"="2010", "Airport"="Stavanger Airport", "Country"="Norway", "Volume"="3674816", "Change"="1.57"}, {"Year"="2010", "Airport"="Bordeaux - Mérignac Airport", "Country"="France", "Volume"="3663702", "Change"="10.42"}, {"Year"="2010", "Airport"="Rhodes International Airport", "Country"="Greece", "Volume"="3586572", "Change"="3.36"}, {"Year"="2010", "Airport"="Turin Airport", "Country"="Italy", "Volume"="3552519", "Change"="10.31"}, {"Year"="2010", "Airport"="Trondheim Airport", "Country"="Norway", "Volume"="3521734", "Change"="2.83"}, {"Year"="2010", "Airport"="Frankfurt-Hahn Airport", "Country"="Germany", "Volume"="3493451", "Change"="-7.91"}, {"Year"="2010", "Airport"="Cagliari-Elmas Airport", "Country"="Italy", "Volume"="3438298", "Change"="3.28"}, {"Year"="2010", "Airport"="Bari Airport", "Country"="Italy", "Volume"="3398110", "Change"="20.27"}]  # Pre-parsed results
    }
  }
  "Data to put into Database" <- w22
  n13 = call "FTW-SQLite-ExecuteScript.vi"("SQLite Connector"=w29, "SQL Script"=w28, "error in"=w30) -> ("SQLite Connector out"=w16:refnum<class "FTW-SQLite-Connector.lvclass">, "error out"=w15:errorcluster)  [unwired: 10 in, 1 out]
  n14 = xnode "FTW-SQLite-Insert.xnode"("SQLite Connector"=w16, "SQL Script"=w23, "Data to Insert"=w22, "error in"=w15) -> ("SQLite Connector out"=w21:refnum<class "FTW-SQLite-Connector.lvclass">, "error out"=w20:errorcluster)  [unwired: 1 out]
  n15 = xnode "FTW-SQLite-Fetch.xnode"("SQLite Connector"=w21, "SQL Script"=w10, "Row Datatype"=T4 {"Year"=0, "Airport"="", "Country"="", "Passengers"=0, "Change"=0.0}, "error in"=w20) -> ("SQLite Connector out"=w14:refnum<class "FTW-SQLite-Connector.lvclass">, "Result Set"=w18:T1, "error out"=w12:errorcluster)  [unwired: 1 out]
  "Results from Database" <- w18
  n16 = xnode "FTW-SQLite-Fetch.xnode"("SQLite Connector"=w14, "SQL Script"=w10, "Row Datatype"=T3 {"Year"="", "Airport"="", "Country"="", "Volume"="", "Change"=""}, "error in"=w12) -> ("SQLite Connector out"=w13:refnum<class "FTW-SQLite-Connector.lvclass">, "Result Set"=w8:T2, "error out"=w11:errorcluster)  [unwired: 1 out]
  n17 = call "FTW-SQLite-CloseConnection.vi"("SQLite Connector"=w13, "error in"=w11) -> ("error out"=w24:errorcluster)  [unwired: 13 in]
  n18 = for {
    tunnel: w18 -> [w75] mode=indexing
    tunnel: "%04d\t%s\t%s\t%d\t%.2f%%\n" ("format string") -> [w69]
    tunnel: [w68] -> w26 mode=indexing
    tunnel: w8 -> [w61] mode=indexing
    tunnel: [w67] -> w7 mode=indexing
    tunnel: "%s\t%s\t%s\t%s\t%s%%\n" ("format string") -> [w60]
    n19 = Unbundle(w61) -> ("Year"=w62:string, "Airport"=w63:string, "Country"=w64:string, "Volume"=w65:string, "Change"=w66:string)
    n20 = Unbundle(w75) -> ("Year"=w74:i32, "Airport"=w73:string, "Country"=w72:string, "Passengers"=w71:i32, "Change"=w70:dbl)
    n21 = Format Into String(format string=w60, w62, w63, w64, w65, w66) -> (resulting string=w67:string)  [unwired: 2 in, 1 out]
    n22 = Format Into String(format string=w69, w74, w73, w72, w71, w70) -> (resulting string=w68:string)  [unwired: 2 in, 1 out]
  }
  n23 = Concatenate Strings(w7) -> (w6:string)
  n24 = Concatenate Strings(w26) -> (w25:string)
  n25 = Equal?(x=w6, y=w2) -> (x = y?=w5:bool)
  n26 = Equal?(x=w25, y=w2) -> (x = y?=w4:bool)
  n27 = And(x=w5, y=w4) -> (x .and. y?=w3:bool)
  n28 = call "FTW-ERR-Assert-Truthy.vi"("Expected Truthy"=w3, "error in"=w24) -> ("error out"=→"Test Result":errorcluster)  [unwired: 13 in]
